vi "GUI_CapillaryDischarge.vi"() -> ()   [LabVIEW 2020]
uses:
  Shared/GUI_Template/GUI_master/tcp_new_data_event.ctl
  Shared/GUI_Template/GUI_master/tcp new data cluster.ctl
  timer.ctl
  <vilib>/Waveform/WDTOps.llb/WDT Waveform Duration DBL.vi
panel:
  in  "GUIdevice 10":string="SRS0"
  in  "time offsets":dbl[](array[numeric])=[0.0, 3e-09, 6e-08, 1.07e-07] format="%#_6p"
  in  "GUIdevice 9":string="Offsets-Timing"
  in  "Trigger on":bool caption="Discharge on"
  in  "GUIdevice 7":string="HeatHighlandT564"
  in  "Tab Control 2":T1(tab)
  out "all traces":waveform(dbl)[](graph)
  in  "value6::9":dbl=1.07e-07 caption="Dischage output" min=-9999999.0 max=9999999.0 step=1e-09 format="%#_6p"
  in  "value5::9":dbl=6e-08 caption="Dischage input" min=-9999999.0 max=9999999.0 step=1e-09 format="%#_6p"
  in  "value4::9":dbl=3e-09 caption="800nm diode" min=-9999999.0 max=9999999.0 step=1e-09 format="%#_6p"
  in  "value3::9":dbl caption="532nm diode" min=-9999999.0 max=9999999.0 step=1e-09 format="%#_6p"
  in  "Digitizer Traces":T2 caption="Digitizer Traces DAQ3 ch0 Timing diode Ch1 Discharge High"
  in  "Enable cap interlock move out":bool
  in  "Force button visibility":bool=TRUE
  in  "amplitude.Channel_C::10":dbl caption="Trigger voltage (0.1 off 1.2 on)" min=-3.0 max=4.0 step=1e-09 format="%#.2f"
  in  "Tab Control":enum32{"Settings for start button", "timeout"}(tab)
  in  "Set Pressure":dbl=30.0 caption="Timer 1 Value" min=0.0 max=100.0
  in  "Set Voltage":dbl=20.0 caption="Timer 1 Value" min=0.0 max=100.0
  in  "Start/Stop discharge":bool
  in  "Pressure Timeout":dbl=10.0 caption="Timer 1 Value" min=0.0 max=100.0
  in  "Voltage Timeout":dbl=10.0 caption="Timer 1 Value" min=0.0 max=100.0
  in  "slaveenable::1":bool
  out "pressure2::2":dbl caption="PDR UP (Torr)" min=-100.0 max=500.0
  in  "SlaveValue::1":dbl caption="Slave %" min=0.0 max=200.0
  out "Data.Channel 2::8":dbl caption="Flow UP (sccm)" min=0.0 max=1000.0
  out "Data.Channel 1::8":dbl caption="Flow Down (sccm)" min=0.0 max=1000.0
  in  "Data.Channel 2::1":dbl caption="PR4000 UP (Torr)" min=0.0 max=1000.0
  in  "GUIdevice 8":string="PL1-PresCtrl-Low2"
  out "Time Elasped Pressure 2":dbl
  out "Time Elasped Voltage 2":dbl
  out "Time Elasped Trig 2":dbl
  out "duration":dbl format="%.2p"
  in  "position::6":enum16{"out", "in", "Unknown"}(ring) caption="POSITION"
  in  "GUIdevice 6":string="PL1-Stage-Cap"
  in  "GUIdevice 5":string="LeCroy8104MS"
  in  "Simulate Trig Level":dbl
  out "Time Elasped Trig":dbl
  in  "Trigger Timeout":dbl=5.0 caption="Timer 1 Value" min=0.0 max=100.0
  in  "Set Trigger Level":dbl=4.0 caption="Timer 1 Value" min=0.0 max=100.0
  in  "GUIdevice 4":string="BellaSRS2"
  out "Discharge Status Msg":string
  out "Time Elasped Voltage":dbl
  in  "Simulate voltage":dbl
  in  "Simulate Pressure read":dbl
  in  "Simulate Pressure write":dbl
  in  "Simulate":bool
  out "Time Elasped Pressure":dbl
  out "pressure::2":dbl caption="PDR Down (Torr)" min=-100.0 max=500.0
  in  "voltage::3":dbl caption="Voltage (kV)" min=0.0 max=40.0
  out "Display Message":string
  in  "Data.Channel 1::1":dbl caption="PR4000 Down (Torr)" min=0.0 max=1000.0
  in  "GUIdevice 3":string="PL1-GlassmanHV"
  in  "GUIdevice 2":string="BELLA_PDR2000"
  in  "GUIdevice 1":string="PL1-PresCtrl-Low1"
  in  "stop":bool
  out "tcp data event":T3
  out "error IO 2":errorcluster
  # "CAPILLARY DISCHARGE CONTROL"
  # "CAPSTAGE"
  # "Check before moving capstage in\n1) pressure\n2) volts\n3) triggers\n4) discharge current"
  # "Diagnostics"
  # "Turn off procedure:\n1) reduce trigger level to 0.5\n2) reduce voltage to 0\n3) reduce pressure to 0"
  # "time offsets"
  # "start/stop needs testing. If doesn't work,\nuse controls on left"
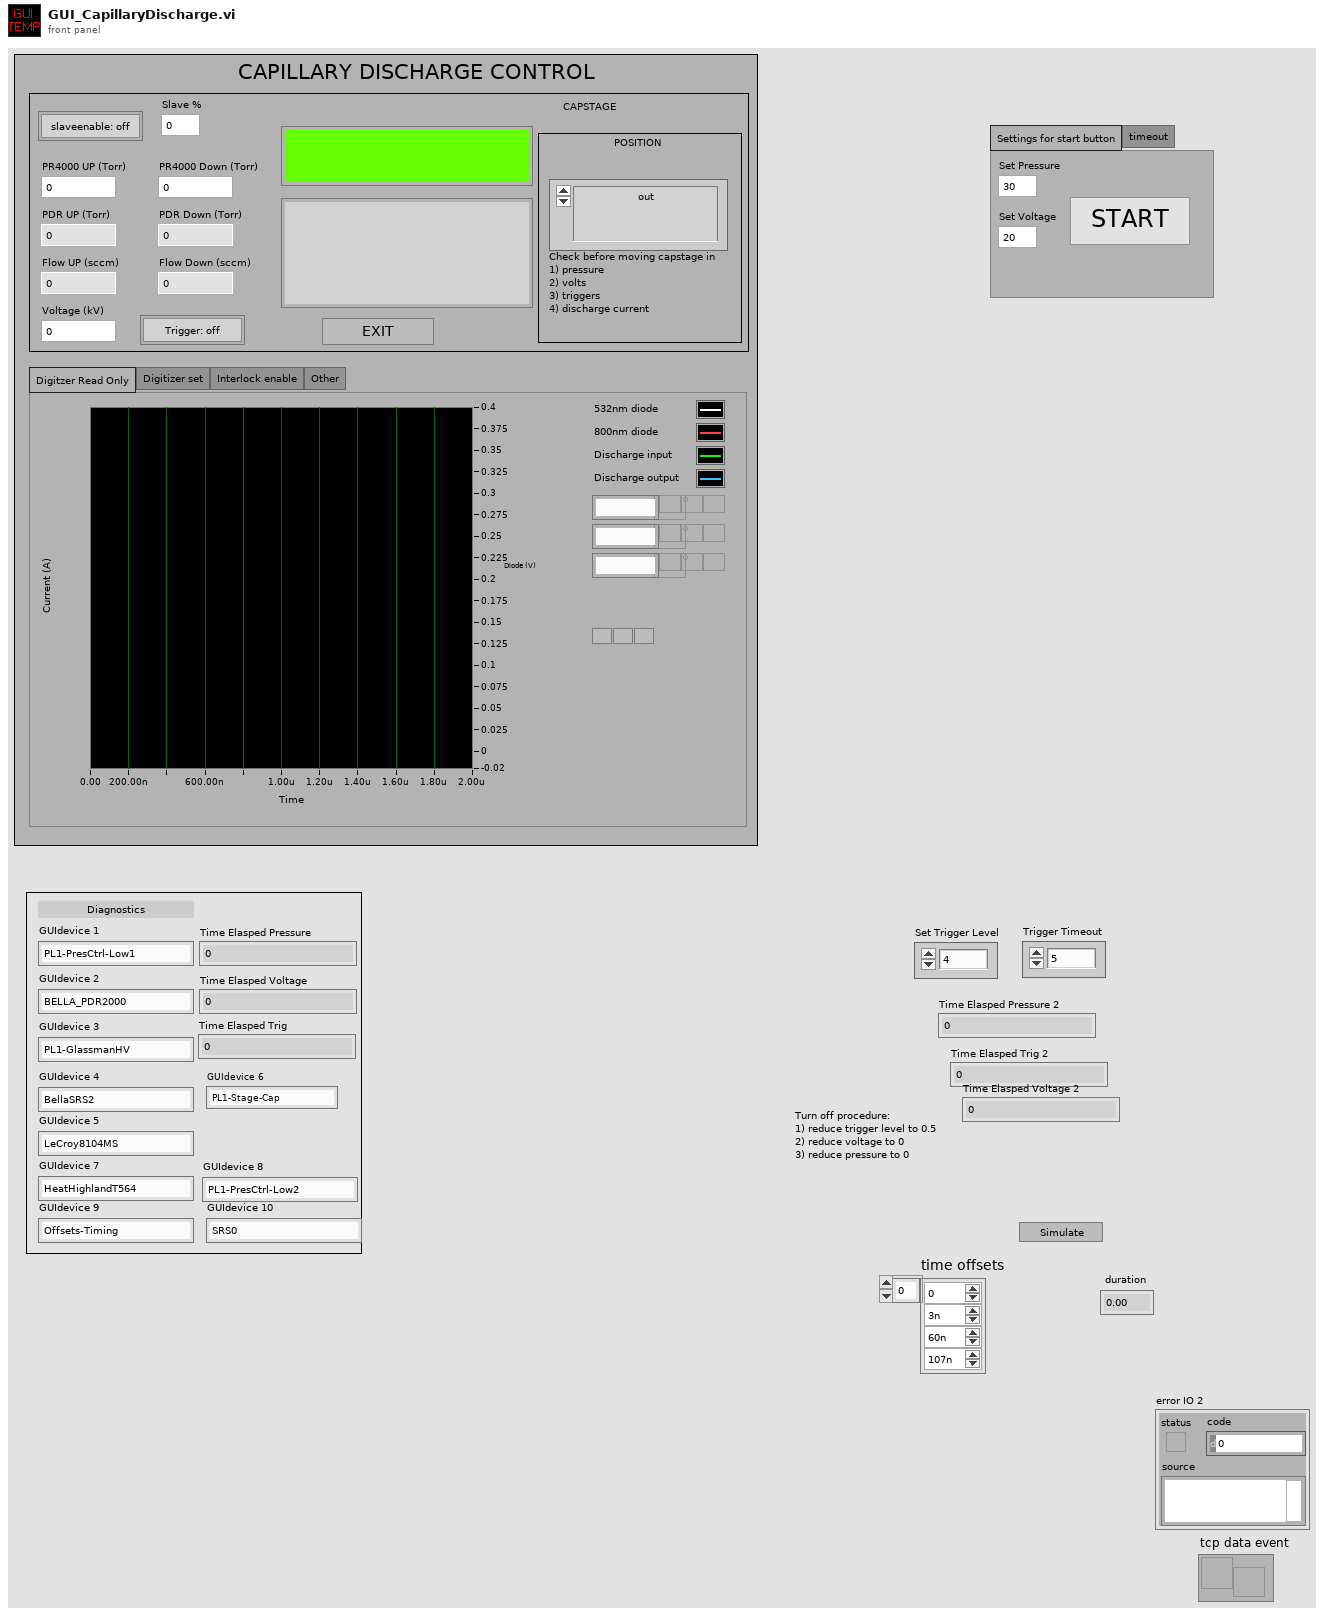
[diagram p1: front panel]
types:
  T1 = enum32{"Digitzer Read Only", "Digitizer set", "Interlock enable", "Other"}
  T2 = cluster{"Channel::5":enum16{"Channel0", "Channel1", "Channel2", "Channel3"}, "scopeTraceGUI::5":waveform(dbl)[]}
  T3 = typedef "tcp_new_data_event.ctl" = refnum<user-event>
  T4 = typedef "tcp new data cluster.ctl" = cluster{"EventEnum":enum16{"new data", "connection status update"}, "Device name":string}
  T5 = enum32{"invalid app kind", "Development System", "Run Time System", "Student Edition", "Embedded LabVIEW", "Evaluation", "Custom"}
  T6 = enum32{"Invalid", "Standard", "Closed", "Hidden", "Minimized", "Maximized"}
  T7 = typedef "timer.ctl" = enum16{"Start", "Read"}
  T8 = cluster{"Core":cluster{"Current VI Reference":refnum<vi>, "Close Panel on Exit?":bool}, "Pressure Timer":bool, "Voltage Timer":bool, "Pressure Timeout":dbl, "Voltage Timeout":dbl, "Display Message":string, "Simulate":bool, "Trigger Timeout":dbl, "Trigger Timer":bool, "Discharge Status Msg":string, "scopeTraceGUI::5":waveform(dbl)[], "scopeTraceGUI::7":waveform(dbl)[]}
  T9 = cluster{"Current VI Reference":refnum<vi>, "Close Panel on Exit?":bool}
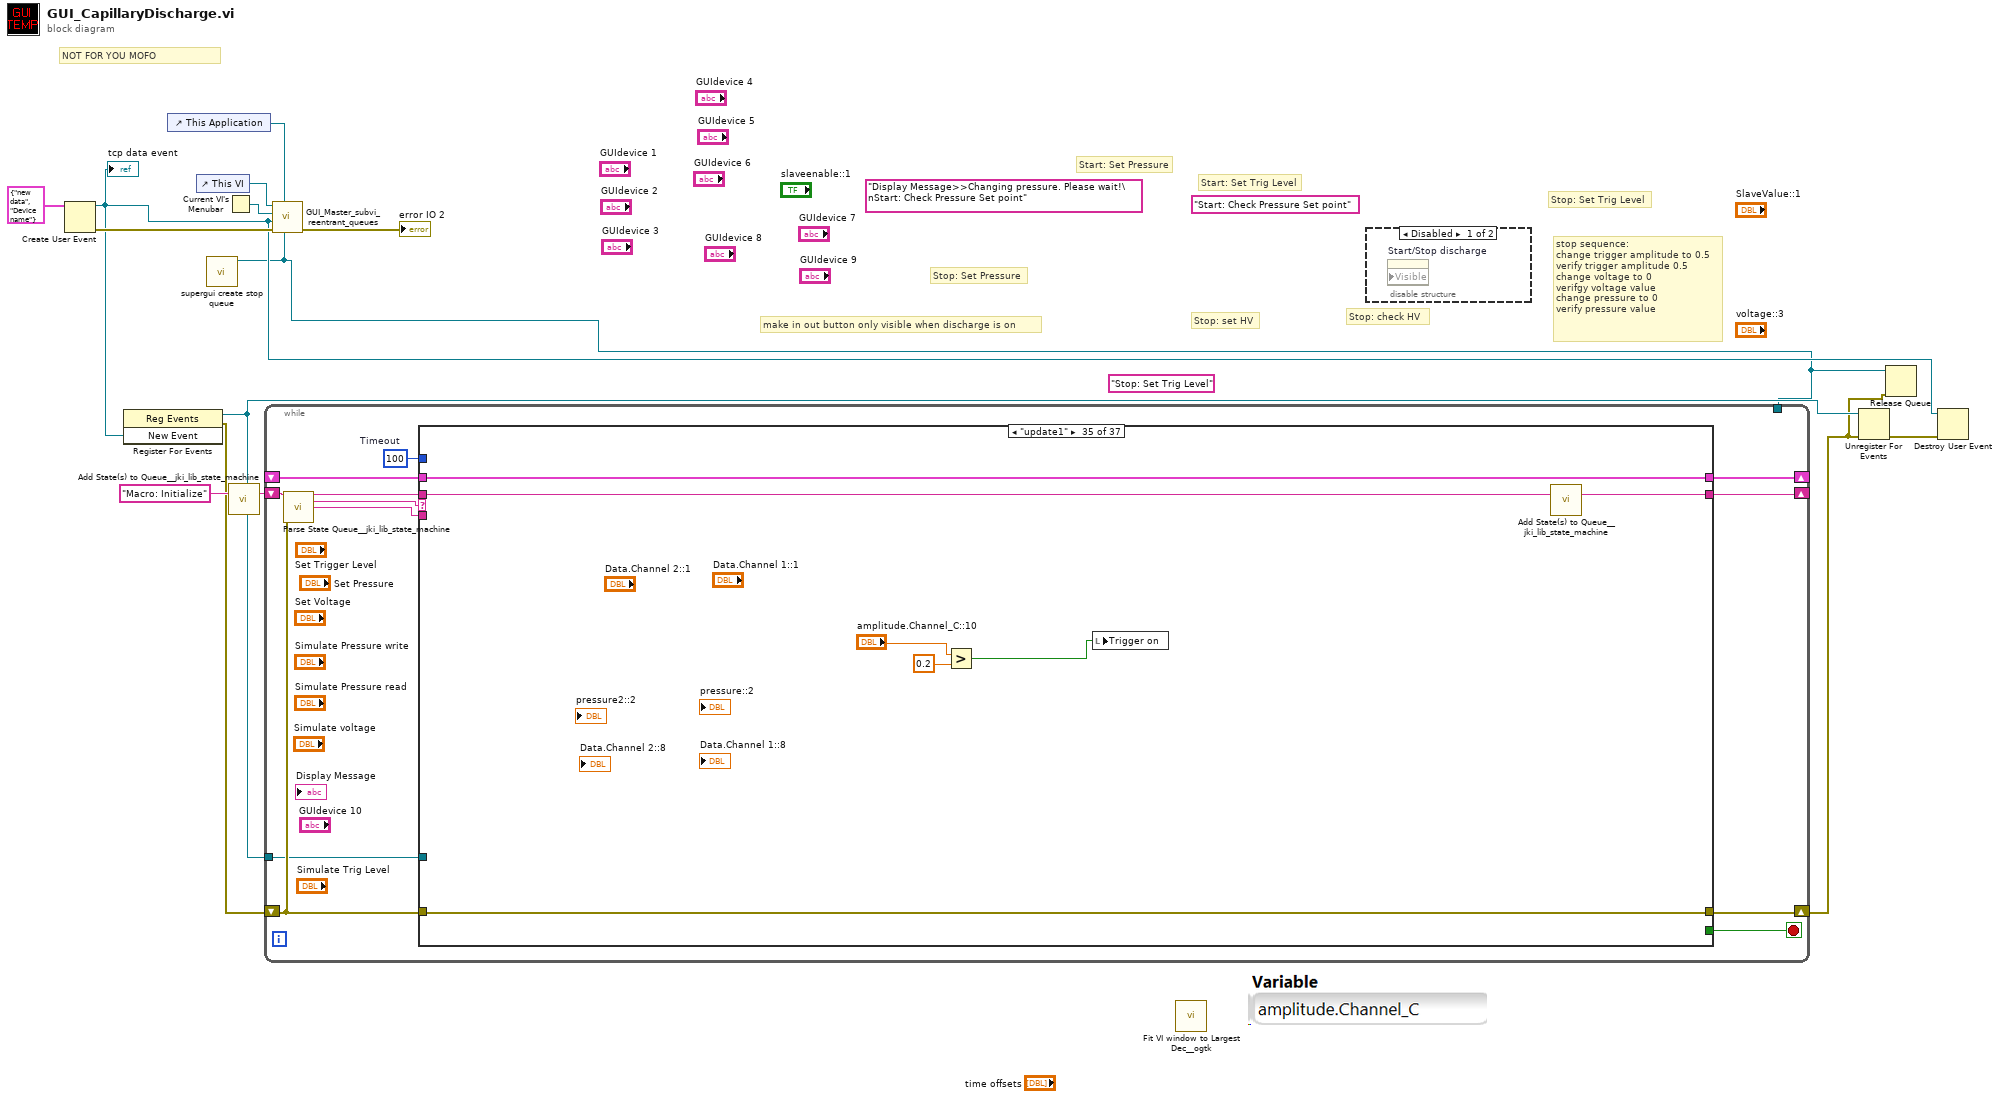
[diagram p0: block diagram]
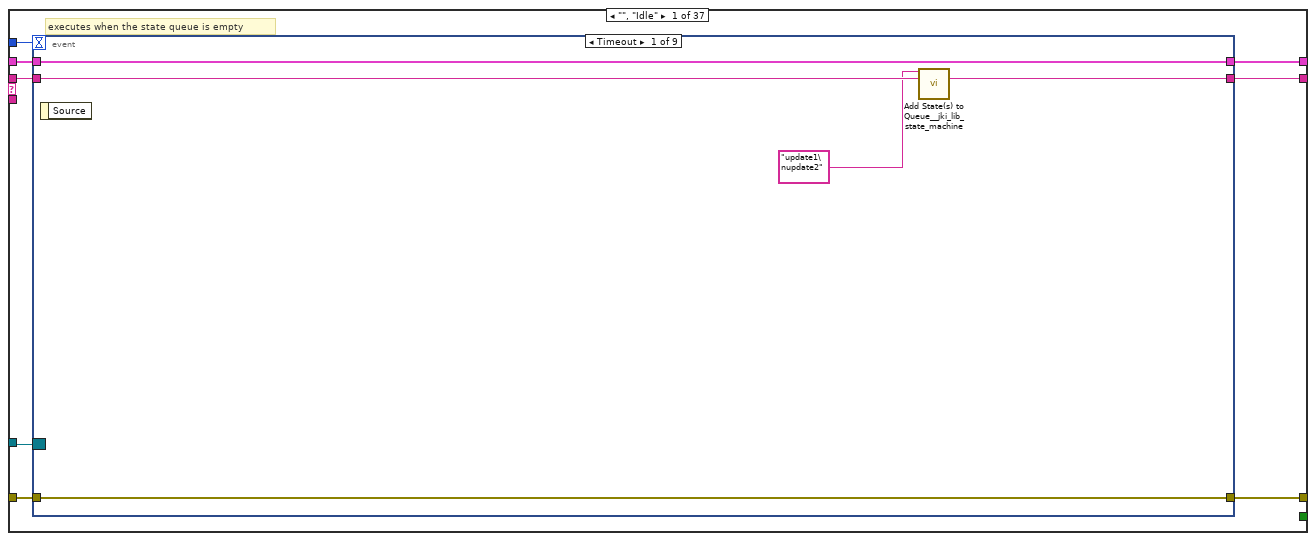
[diagram p3: hidden frame]
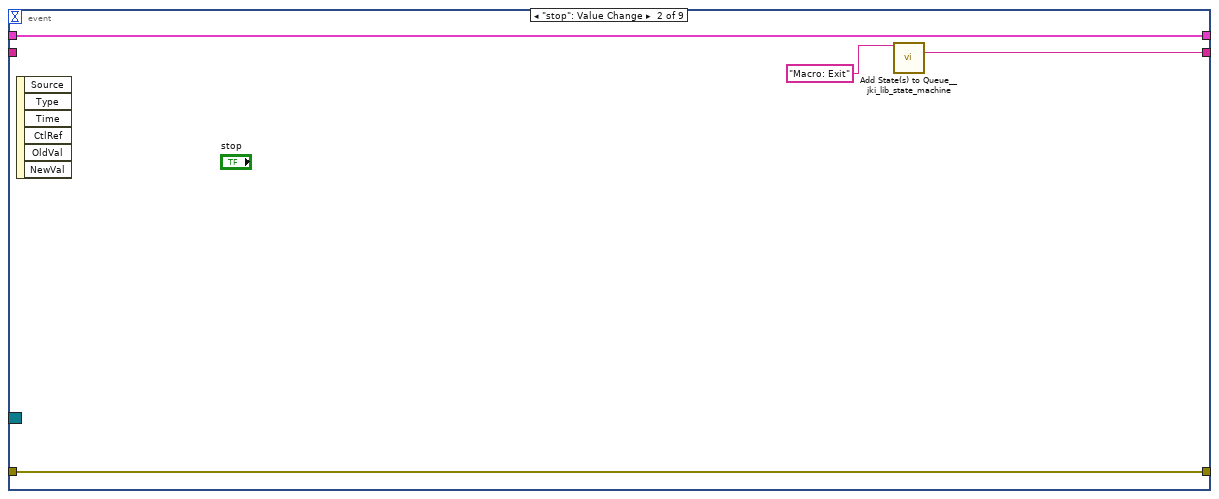
[diagram p4: hidden frame]
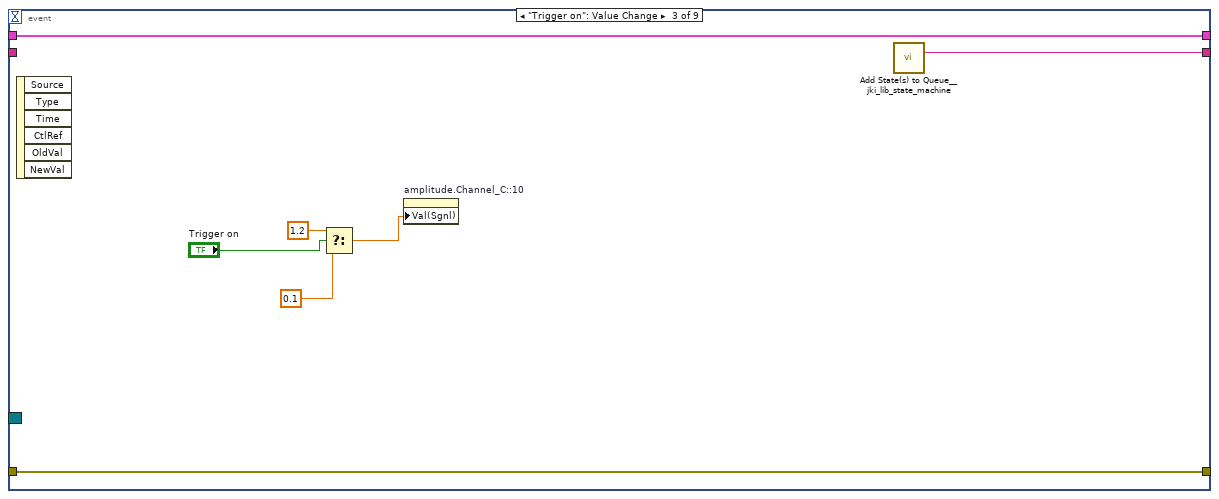
[diagram p5: hidden frame]
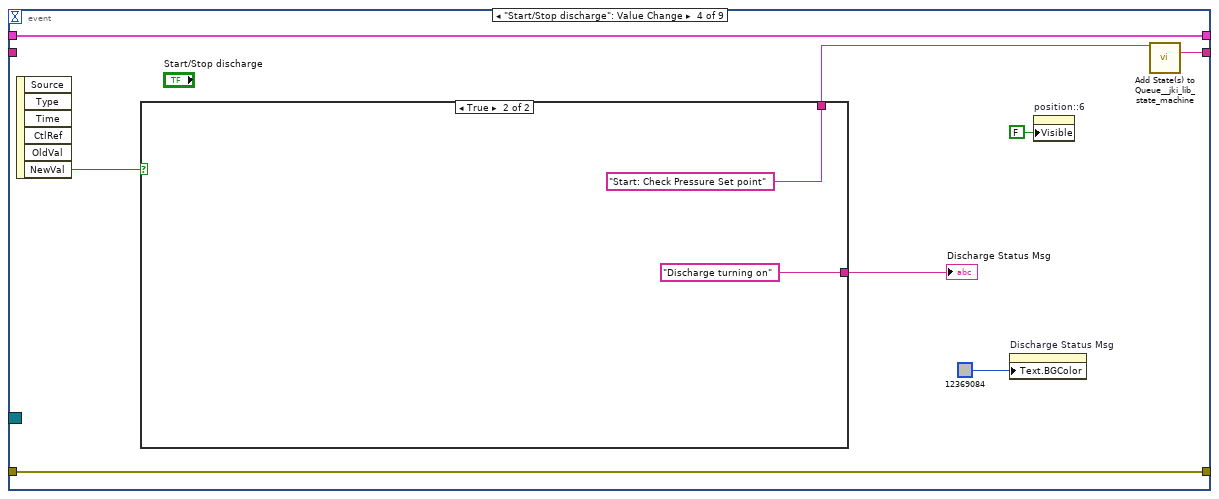
[diagram p6: hidden frame]
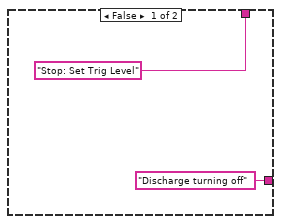
[diagram p7: hidden frame]
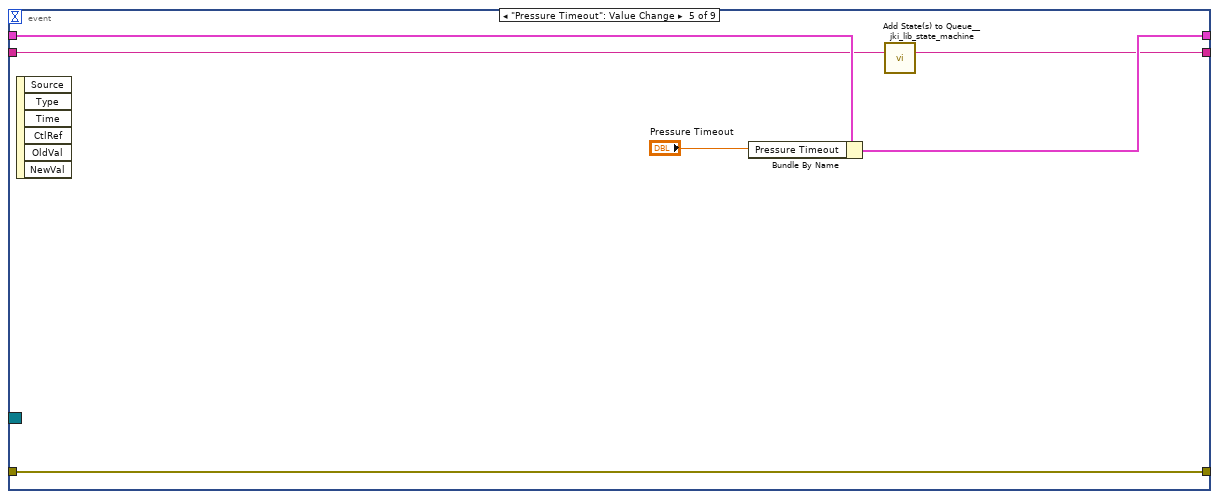
[diagram p8: hidden frame]
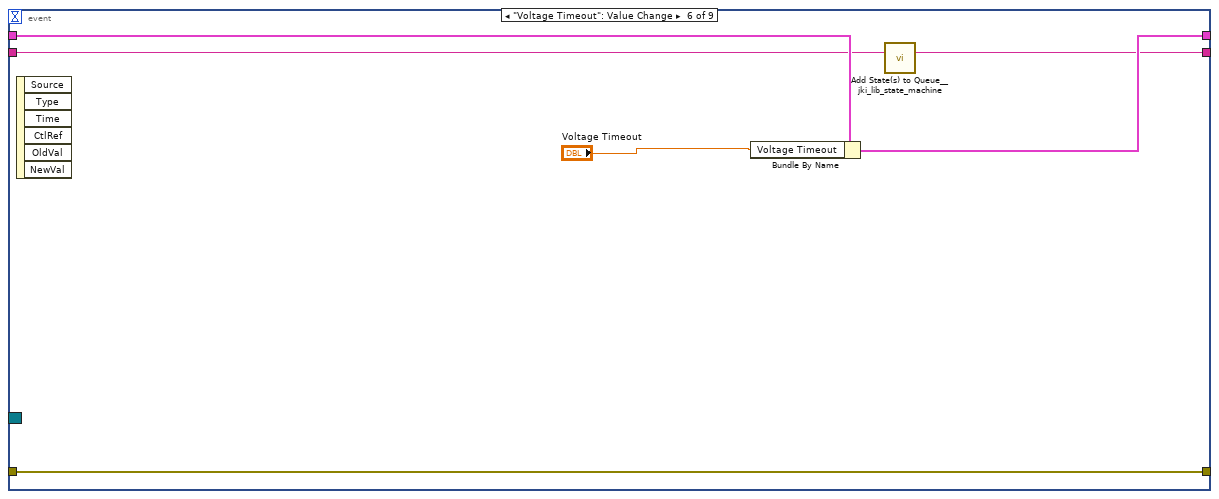
[diagram p9: hidden frame]
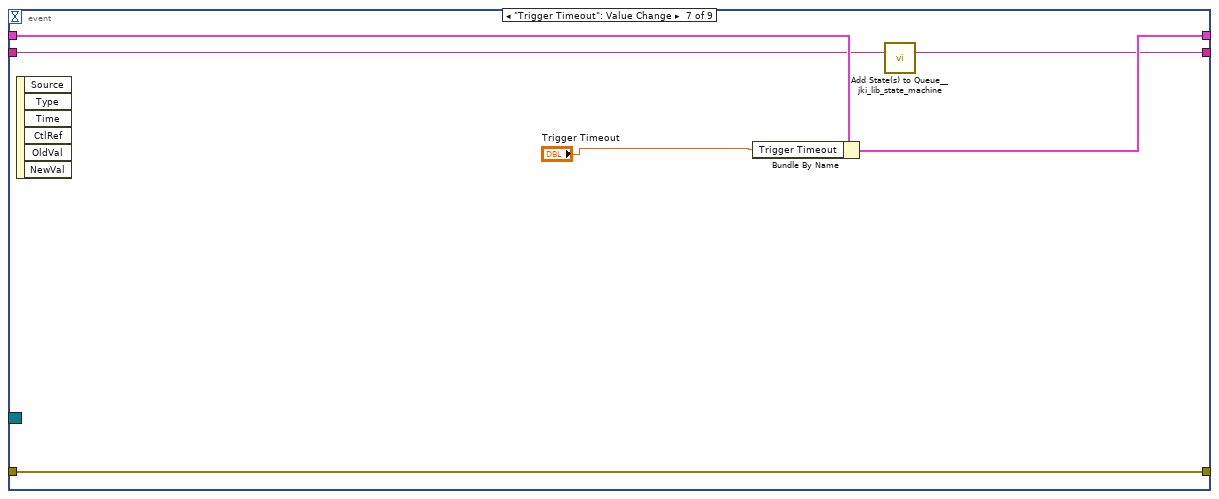
[diagram p10: hidden frame]
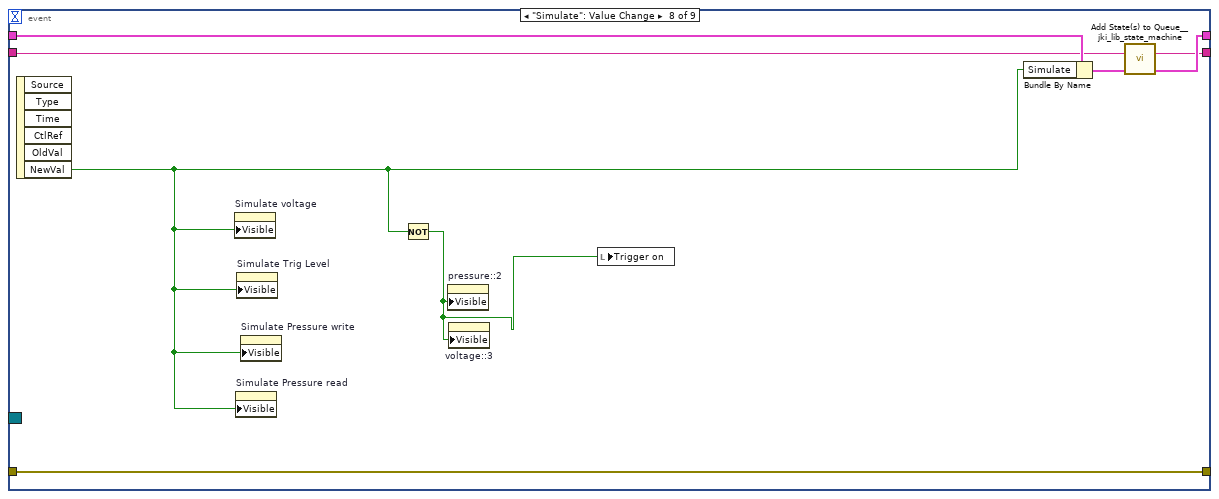
[diagram p11: hidden frame]
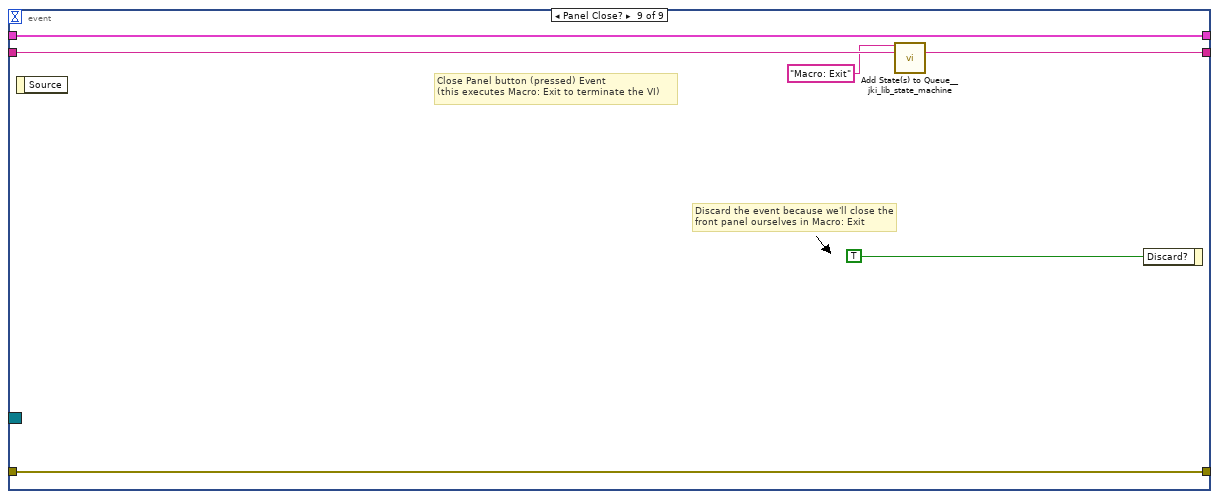
[diagram p12: hidden frame]
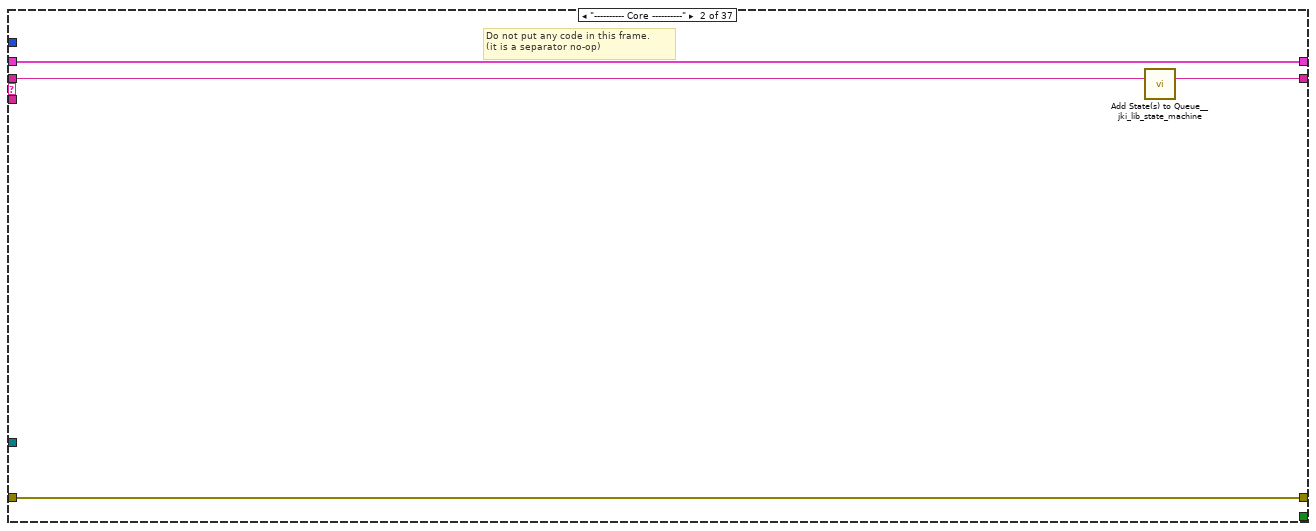
[diagram p13: hidden frame]
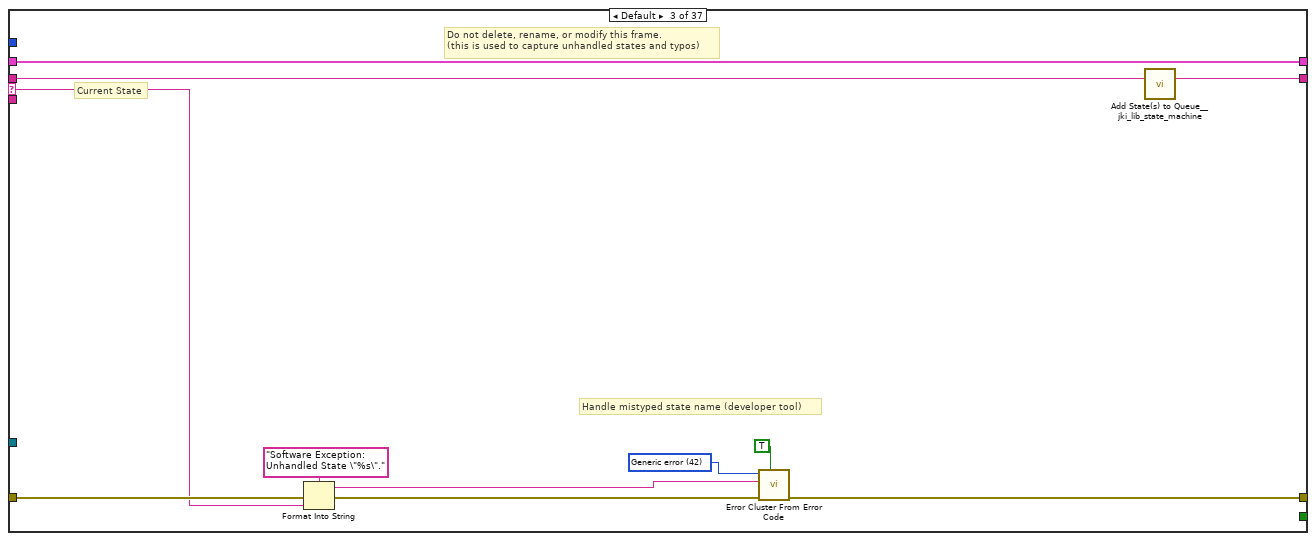
[diagram p14: hidden frame]
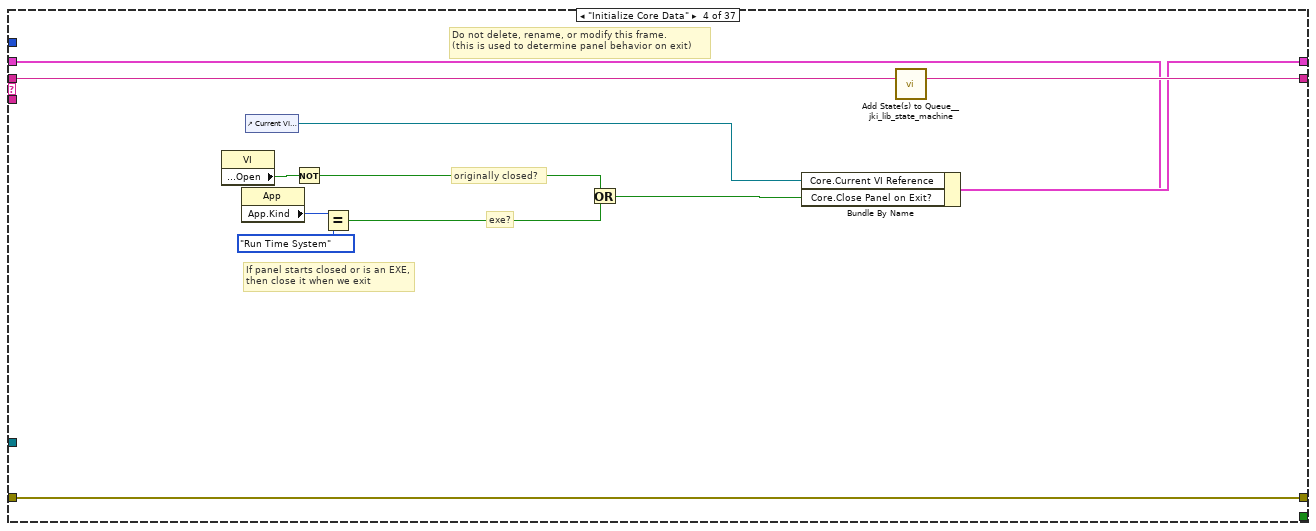
[diagram p15: hidden frame]
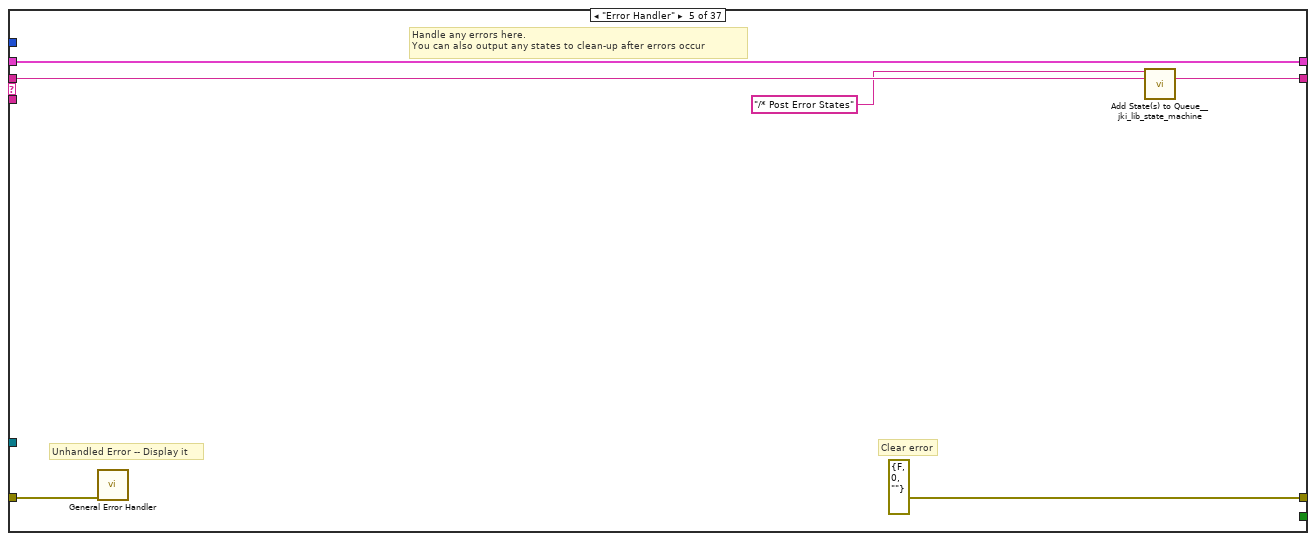
[diagram p16: hidden frame]
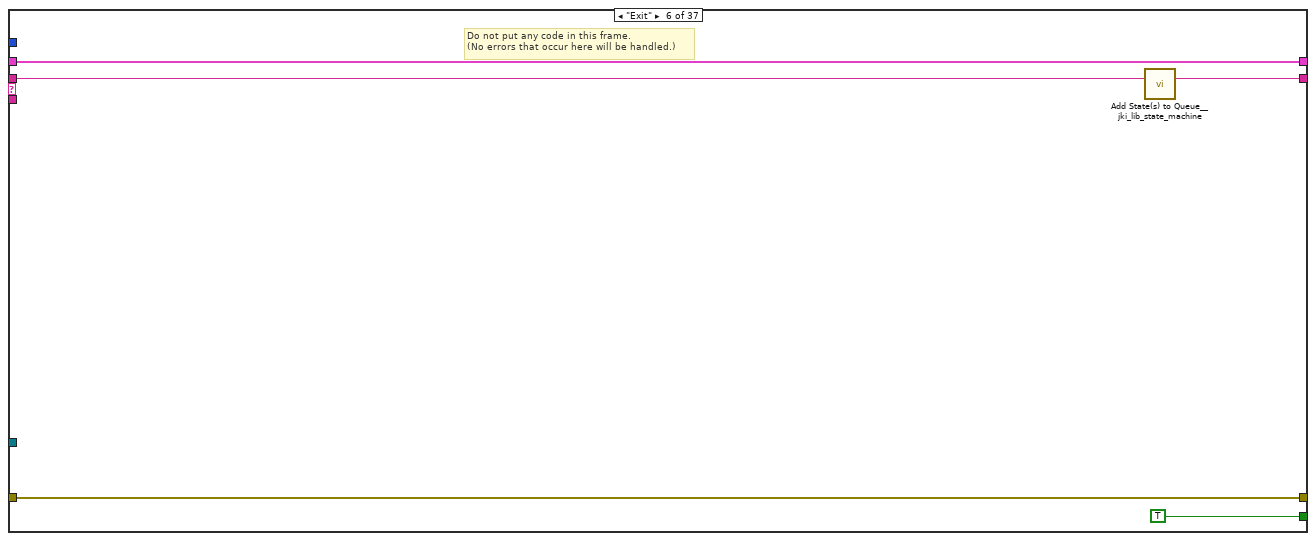
[diagram p17: hidden frame]
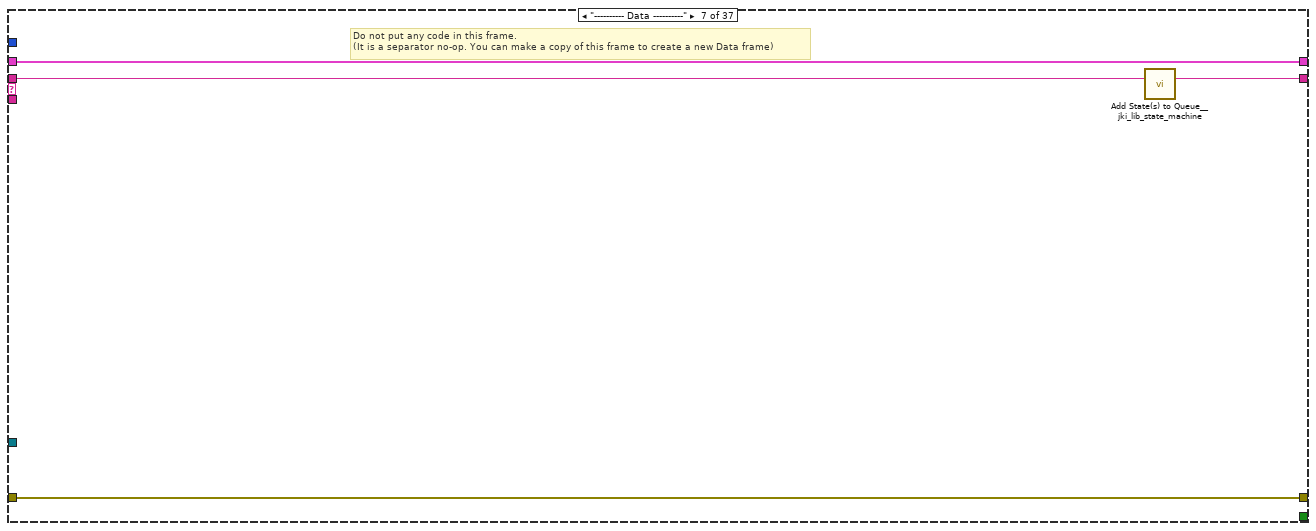
[diagram p18: hidden frame]
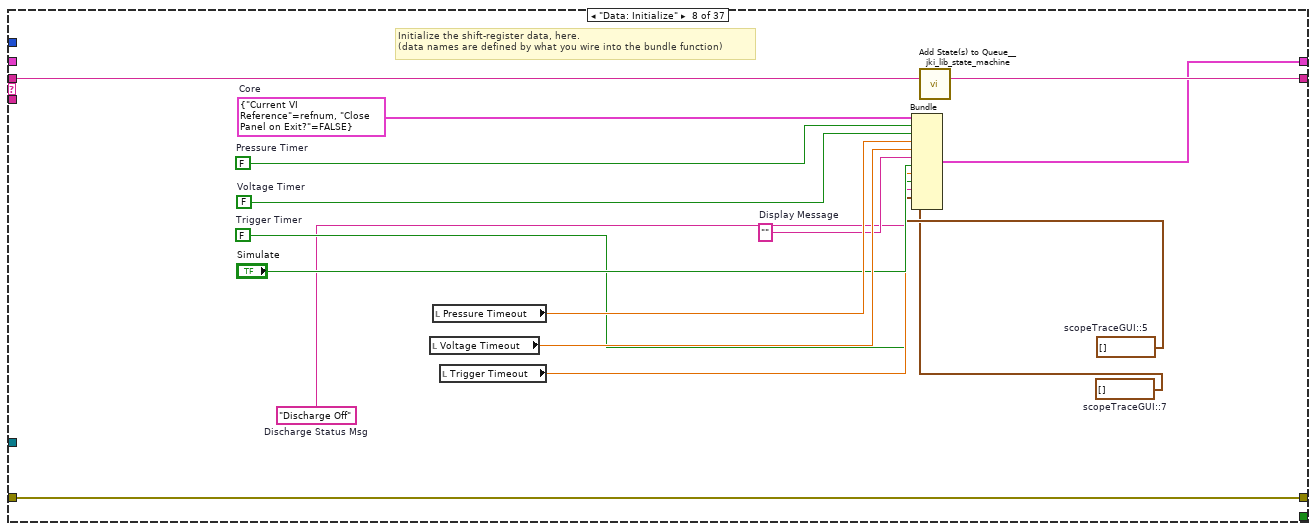
[diagram p19: hidden frame]
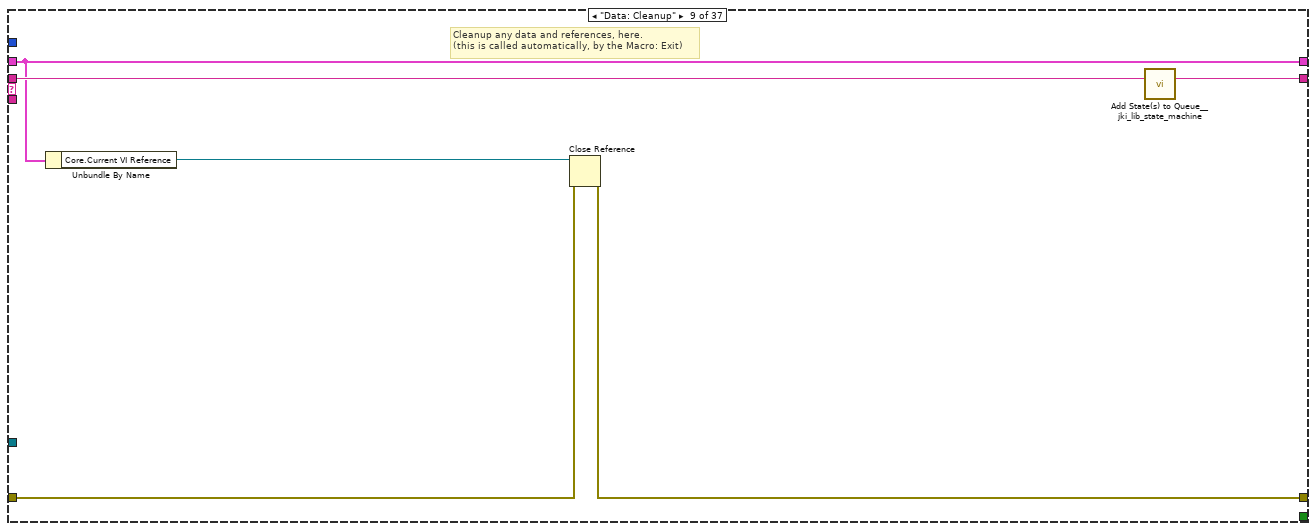
[diagram p20: hidden frame]
diagram:
  (unwired) "Stop: Set Trig Level"
  (unwired) "Start: Check Pressure Set point"
  (unwired) "Display Message>>Changing pressure. Please wait!\nStart: Check Pressure Set point" ("State(s) in Front (\"\")")
  # "make in out button only visible when discharge is on"
  # "Stop: Set Pressure"
  # "Stop: check HV"
  # "Stop: set HV"
  # "Stop: Set Trig Level"
  # "stop sequence:\nchange trigger amplitude to 0.5\nverify trigger amplitude 0.5\nchange voltage to 0\nverifgy voltage value\nchange pressure to 0\nverify pressure value"
  # "Start: Set Pressure"
  # "Start: Set Trig Level"
  # "NOT FOR YOU MOFO"
  n1 = Create User Event(user event datatype=T4 {"EventEnum"=enum."new data", "Device name"="Device name"} ("New Event")) -> (user event=w8:refnum<user-event>, error out=w10:errorcluster)  [unwired: 1 in]
  "tcp data event" <- w8
  n2 = register-events(w8) -> (reference out=w4:refnum<event-registration>, error out=w5:errorcluster)  [unwired: 2 in]
  n3 = control-ref of="This Application"() -> (w9:refnum<vi>)
  n4 = control-ref of="This VI"() -> (w13:refnum<vi>)
  n5 = call "supergui create stop queue.vi"() -> ("STOP Queue out"=w3:refnum<queue>)  [unwired: 11 in]
  n6 = Current VI's Menubar() -> (w12:refnum<k9>)
  n7 = call <vilib>:"Add State(s) to Queue__jki_lib_state_machine.vi"("State(s) in (\"\")"="Macro: Initialize") -> ("States Out"=w7:string)  [unwired: 14 in]
  n8 = while "JKI - String-Based Queued State Machine (Basic) v1.0" {
    shift-right: [w19] -> _
    shift-left: _ -> [w18]
    shift-right: [w22] -> w1
    shift-left: w5 -> [w16]
    shift-right: [w21] -> _
    shift-left: w7 -> [w23]
    tunnel: w4 -> [w15]
    tunnel: w3 -> [_]
    stop <- w20 stop-if-true
    w17 = 100  # Timeout
    n9 = call <vilib>:"Parse State Queue__jki_lib_state_machine.vi"("State Queue"=w23, "Error In (no error)"=w16) -> ("Remaining States"=w25:string, "Current State"=w26:string, "Arguments"=w24:string)  [unwired: 11 in]
    n10 = case shown="\"update1\"" w26 {
      selector: w26 -> [_ _ w98 _ _ _ _ _ _ _ _ _ _ _ _ _ _ _ _ _ _ _ _ _ _ _ _ _ _ _ _ _ _ _ _ _ _]
      tunnel: w25 -> [w34 w97 w102 w120 w126 w131 w135 w151 w157 w161 w167 w177 w188 w214 w219 w229 w233 w242 w277 w305 w318 w329 w367 w395 w409 w417 w440 w462 w473 w485 w491 w497 w504 w540 w581 w585 w599]
      tunnel: w24 -> [_ _ _ _ _ _ _ _ _ _ _ w172 w182 _ _ _ _ _ _ _ _ _ _ _ _ _ _ _ _ _ _ _ w500 _ _ _ _]
      tunnel: w18 -> [w32 w94 w100 w111 w123 w129 w132 _ w152 w158 w163 w175 w184 w211 w216 w227 w230 w237 w272 w299 w312 w322 w361 w389 w403 w416 w439 w460 w471 w482 w488 w494 w498 w507 w578 w582 w594]
      tunnel: [w31 w95 w104 w117 errorcluster {"status"=FALSE, "code"=0, "source"=""} ("error out") w128 w133 w148 w153 w159 w165 w173 w185 w212 w217 w220 w231 w240 w275 w303 w316 w327 w365 w393 w407 w413 w436 w458 w469 w483 w489 w495 w502 w538 w579 w583 w586] -> w22
      tunnel: w16 -> [w30 w95 w103 w117 w122 w128 w133 w148 w154 w159 w165 w174 w186 w212 w217 w220 w231 w240 w275 w303 w316 w327 w365 w393 w407 w413 w436 w458 w469 w483 w489 w495 w502 w538 w579 w583 w587]
      tunnel: [w33 w96 w101 w119 w125 w130 w134 w150 w156 w160 w166 w176 w187 w213 w218 w228 w232 w241 w276 w304 w317 w328 w366 w394 w408 w414 w437 w461 w472 w484 w490 w496 w503 w539 w580 w584 w598] -> w21
      tunnel: [_ _ _ _ _ TRUE _ _ _ _ _ _ _ _ _ _ _ _ _ _ _ _ _ _ _ _ _ _ _ _ _ _ _ _ _ _ _] -> w20
      tunnel: [w29 w94 w100 w118 w123 w129 w132 w149 w152 w158 w163 w175 w184 w211 w216 w227 w230 w236 w271 w301 w314 w321 w360 w391 w405 w415 w438 w459 w470 w481 w487 w493 w498 w507 w578 w582 w596] -> w19
      tunnel: w17 -> [w28 _ _ _ _ _ _ _ _ _ _ _ _ _ _ _ _ _ _ _ _ _ _ _ _ _ _ _ _ _ _ _ _ _ _ _ _]
      tunnel: w15 -> [w27 _ _ _ _ _ _ _ _ _ _ _ _ _ _ _ _ _ _ _ _ _ _ _ _ _ _ _ _ _ _ _ _ _ _ _ _]
      frame "", "Idle" {
        # "executes when the state queue is empty"
        n11 = event shown="[0] Timeout" {
          selector: w27 -> [_ _ _ _ _ _ _ _ _]
          dyn-events: _ -> [_ _ _ _ _ _ _ _ _]
          timeout: w28 -> [_ _ _ _ _ _ _ _ _]
          tunnel: w34 -> [w39 _ _ _ w64 w71 w77 w83 w93]
          tunnel: [w38 w41 w49 w57 w63 w70 w76 w84 w92] -> w33
          tunnel: w32 -> [w36 w43 w50 w58 w67 w73 w79 w87 w90]
          tunnel: [w37 w40 w48 w56 w68 w74 w80 w85 w91] -> w31
          tunnel: w30 -> [w37 w40 w48 w56 w68 w74 w80 w85 w91]
          tunnel: [w36 w43 w50 w58 w66 w72 w78 w86 w90] -> w29
          event Timeout {
            n12 = event-data() -> ()  [unwired: 1 in, 1 out]
            n13 = call <vilib>:"Add State(s) to Queue__jki_lib_state_machine.vi"("State(s) in Front (\"\")"="update1\nupdate2" ("State(s) in Front (\"\")"), "State(s) in (\"\")"=w39) -> ("States Out"=w38:string)  [unwired: 13 in]
          }
          event "stop": Value Change {
            n14 = event-data() -> ()  [unwired: 1 in, 6 out]
            n15 = call <vilib>:"Add State(s) to Queue__jki_lib_state_machine.vi"("State(s) in Front (\"\")"="Macro: Exit") -> ("States Out"=w41:string)  [unwired: 14 in]
          }
          event "Trigger on": Value Change {
            n16 = event-data() -> ()  [unwired: 1 in, 6 out]
            n17 = Select(t=1.2, s="Trigger on", f=0.1 ("t")) -> (s? t:f=w44:dbl)
            n18 = property on="amplitude.Channel_C::10" class="DigNum (strict)"("Val(Sgnl)"=w44) -> ()  [unwired: 2 in, 2 out]
            n19 = call <vilib>:"Add State(s) to Queue__jki_lib_state_machine.vi"() -> ("States Out"=w49:string)  [unwired: 15 in]
          }
          event "Start/Stop discharge": Value Change {
            n20 = event-data() -> ("NewVal"=w55:bool)  [unwired: 1 in, 5 out]
            n21 = case shown="True" w55 {
              tunnel: ["Stop: Set Trig Level" "Start: Check Pressure Set point"] -> w54
              tunnel: ["Discharge turning off" ("Discharge Status Msg") "Discharge turning on" ("Discharge Status Msg")] -> w52
              frame False {
              }
              frame True {
              }
            }
            "Discharge Status Msg" <- w52
            n22 = property on="Discharge Status Msg" class="Str"("Text.BGColor"=u32 12369084) -> ()  [unwired: 2 in, 2 out]
            n23 = property on="position::6" class="Enum (strict)"("Visible"=FALSE) -> ()  [unwired: 2 in, 2 out]
            n24 = call <vilib>:"Add State(s) to Queue__jki_lib_state_machine.vi"("State(s) in Front (\"\")"=w54) -> ("States Out"=w57:string)  [unwired: 14 in]
          }
          event "Pressure Timeout": Value Change {
            n25 = event-data() -> ()  [unwired: 1 in, 6 out]
            n26 = Bundle By Name(cluster=w67, "Pressure Timeout"="Pressure Timeout") -> (w66:T8)
            n27 = call <vilib>:"Add State(s) to Queue__jki_lib_state_machine.vi"("State(s) in (\"\")"=w64) -> ("States Out"=w63:string)  [unwired: 14 in]
          }
          event "Voltage Timeout": Value Change {
            n28 = event-data() -> ()  [unwired: 1 in, 6 out]
            n29 = Bundle By Name(cluster=w73, "Voltage Timeout"="Voltage Timeout") -> (w72:T8)
            n30 = call <vilib>:"Add State(s) to Queue__jki_lib_state_machine.vi"("State(s) in (\"\")"=w71) -> ("States Out"=w70:string)  [unwired: 14 in]
          }
          event "Trigger Timeout": Value Change {
            n31 = event-data() -> ()  [unwired: 1 in, 6 out]
            n32 = Bundle By Name(cluster=w79, "Trigger Timeout"="Trigger Timeout") -> (w78:T8)
            n33 = call <vilib>:"Add State(s) to Queue__jki_lib_state_machine.vi"("State(s) in (\"\")"=w77) -> ("States Out"=w76:string)  [unwired: 14 in]
          }
          event "Simulate": Value Change {
            n34 = event-data() -> ("NewVal"=w82:bool)  [unwired: 1 in, 5 out]
            n35 = property on="Simulate voltage" class="DigNum (strict)"("Visible"=w82) -> ()  [unwired: 2 in, 2 out]
            n36 = property on="Simulate Pressure read" class="DigNum (strict)"("Visible"=w82) -> ()  [unwired: 2 in, 2 out]
            n37 = property on="Simulate Trig Level" class="DigNum (strict)"("Visible"=w82) -> ()  [unwired: 2 in, 2 out]
            n38 = property on="Simulate Pressure write" class="DigNum (strict)"("Visible"=w82) -> ()  [unwired: 2 in, 2 out]
            n39 = Not(x=w82) -> (.not. x?=w81:bool)
            n40 = property on="pressure::2" class="DigNum (strict)"("Visible"=w81) -> ()  [unwired: 2 in, 2 out]
            n41 = property on="voltage::3" class="DigNum (strict)"("Visible"=w81) -> ()  [unwired: 2 in, 2 out]
            n42 = local write "Trigger on"(w81) -> ()
            n43 = Bundle By Name(cluster=w87, "Simulate"=w82) -> (w86:T8)
            n44 = call <vilib>:"Add State(s) to Queue__jki_lib_state_machine.vi"("State(s) in (\"\")"=w83) -> ("States Out"=w84:string)  [unwired: 14 in]
          }
          event Panel Close? {
            # "Discard the event because we'll close the front panel ourselves in Macro: Exit"
            # "Close Panel button (pressed) Event\n(this executes Macro: Exit to terminate the VI)"
            n45 = event-data() -> ()  [unwired: 1 in, 1 out]
            n46 = call <vilib>:"Add State(s) to Queue__jki_lib_state_machine.vi"("State(s) in Front (\"\")"="Macro: Exit", "State(s) in (\"\")"=w93) -> ("States Out"=w92:string)  [unwired: 13 in]
            n47 = event-data("Discard?"=TRUE) -> ()  [unwired: 1 in, 1 out]
          }
        }
      }
      frame "---------- Core ----------" {
        # "Do not put any code in this frame.\n(it is a separator no-op)"
        n48 = call <vilib>:"Add State(s) to Queue__jki_lib_state_machine.vi"("State(s) in (\"\")"=w97) -> ("States Out"=w96:string)  [unwired: 14 in]
      }
      frame Default {
        w107 = 42 items=["No error", "Argument error", "Memory is full", "Out of zone", "End of file", "File already open", "Generic file I/O error", "File not found", "File permission error", "Disk is full", "Duplicate path", "Too many files open", "System feature not enabled", "Resource file not found", "Cannot add resource", "Resource not found", "Image not found", "Image memory error", "Pen does not exist", "Config type invalid", "Config token not found", "Config parse error", "Config memory error", "Bad external code format", "Bad external code offset", "External code not present", "Null window", "Destroy window error", "Null menu", "Print aborted", "Bad print record", "Print driver error", "Windows error during printing", "Memory error during printing", "Print dialog error", "Generic print error", "Invalid device refnum", "Device not found", "Device parameter error", "Device unit error", "Cannot open device", "Device call aborted", "Generic error", "Cancelled by user", "Object ID too low", "Object ID too high", "Object not in heap", "Unknown heap", "Unknown object (invalid DefProc)", "Unknown object (DefProc not in table)", "Message out of range", "Invalid (null) method", "Unknown message", "Manager call not supported", "Bad address", "Network operation in progress", "Network operation timed out", "Connection is busy", "Network attribute not supported", "Network error", "Address in use", "System out of memory", "Connection aborted", "Connection refused", "Not connected", "Already connected", "Connection closed", "Initialization error (interapplication manager)", "Bad occurrence", "Wait on unbound occurrence handler", "Occurrence queue overflow", "Datalog type conflict", "Unused", "Unrecognized type (interapplication manager)", "Memory corrupt", "Failed to make temporary DLL", "Old CIN version", "Drag socket not found", "Failed to load drop-object", "Failed to register OLE object", "Failed to release OLE object", "Format specifier type mismatch", "Unknown format specifier", "Too few format specifiers", "Too many format specifiers", "Scan failed", "Newer CIN version", "Error converting to variant", "Runtime menu error", "Password tampered", "Variant attribute not found", "Incompatible variant data type", "Event data is not available", "Event Store is not present", "Occurrence is not found", "Event Queue is not created", "Event info is not available", "Refnum passed is NULL", "Error retrieving Class GUID", "Error retrieving CoClass GUID", "Error retrieving TypeLib GUID.", "Bad built application magic bytes.", "Specific driver is different from the specific driver associated with the Logical Name.", "There is no session opened to the class driver.", "Max Error", "MAX - Error with config objects", "MAX - Error loading configuration", "MAX - Group not supported"]
        # "Current State"
        # "Do not delete, rename, or modify this frame.\n(this is used to capture unhandled states and typos)"
        # "Handle mistyped state name (developer tool)"
        n49 = Format Into String(format string="Software Exception: Unhandled State \"%s\"." ("message"), error in=w103, w98) -> (resulting string=w106:string, error out=w105:errorcluster)  [unwired: 1 in]
        n50 = call <vilib>:"Error Cluster From Error Code.vi"("show call chain? (False)"=TRUE, "error in (no error)"=w105, "error message (\"\")"=w106, "error code (0)"=w107) -> ("error out"=w104:errorcluster)  [unwired: 5 in]
        n51 = call <vilib>:"Add State(s) to Queue__jki_lib_state_machine.vi"("State(s) in (\"\")"=w102) -> ("States Out"=w101:string)  [unwired: 14 in]
      }
      frame "Initialize Core Data" {
        # "Do not delete, rename, or modify this frame.\n(this is used to determine panel behavior on exit)"
        # "originally closed?"
        # "exe?"
        # "If panel starts closed or is an EXE, then close it when we exit"
        n52 = property class="VI"() -> ("Front Panel.Open"=w116:bool)  [unwired: 2 in, 2 out]
        n53 = property class="App"() -> ("App.Kind"=w115:T5)  [unwired: 2 in, 2 out]
        n54 = control-ref of="Current VI Reference"() -> (w109:refnum<vi>)
        n55 = Not(x=w116) -> (.not. x?=w113:bool)
        n56 = Equal?(x=w115, y=T5."Run Time System" ("Application:Kind")) -> (x = y?=w112:bool)
        n57 = Or(x=w113, y=w112) -> (x .or. y?=w110:bool)
        n58 = Bundle By Name(cluster=w111, "Core.Current VI Reference"=w109, "Core.Close Panel on Exit?"=w110) -> (w118:T8)
        n59 = call <vilib>:"Add State(s) to Queue__jki_lib_state_machine.vi"("State(s) in (\"\")"=w120) -> ("States Out"=w119:string)  [unwired: 14 in]
      }
      frame "Error Handler" {
        # "Unhandled Error -- Display it"
        # "Handle any errors here.\nYou can also output any states to clean-up after errors occur"
        # "Clear error"
        n60 = call <vilib>:"General Error Handler.vi"("error in (no error)"=w122) -> ()  [unwired: 10 in, 5 out]
        n61 = call <vilib>:"Add State(s) to Queue__jki_lib_state_machine.vi"("State(s) in Front (\"\")"="/* Post Error States", "State(s) in (\"\")"=w126) -> ("States Out"=w125:string)  [unwired: 13 in]
      }
      frame "Exit" {
        # "Do not put any code in this frame.\n(No errors that occur here will be handled.)"
        n62 = call <vilib>:"Add State(s) to Queue__jki_lib_state_machine.vi"("State(s) in (\"\")"=w131) -> ("States Out"=w130:string)  [unwired: 14 in]
      }
      frame "---------- Data ----------" {
        # "Do not put any code in this frame.\n(It is a separator no-op. You can make a copy of this frame to create a new Data frame)"
        n63 = call <vilib>:"Add State(s) to Queue__jki_lib_state_machine.vi"("State(s) in (\"\")"=w135) -> ("States Out"=w134:string)  [unwired: 14 in]
      }
      frame "Data: Initialize" {
        w136 = waveform(dbl)[] []  # scopeTraceGUI::7
        w137 = waveform(dbl)[] []  # scopeTraceGUI::5
        w138 = "Discharge Off"  # Discharge Status Msg
        w139 = FALSE  # Trigger Timer
        w142 = ""  # Display Message
        w145 = FALSE  # Voltage Timer
        w146 = T9 {"Current VI Reference"=refnum, "Close Panel on Exit?"=FALSE}  # Core
        w147 = FALSE  # Pressure Timer
        # "Initialize the shift-register data, here.\n(data names are defined by what you wire into the bundle function)"
        n64 = local read "Voltage Timeout"() -> (w143:dbl)
        n65 = local read "Pressure Timeout"() -> (w144:dbl)
        n66 = local read "Trigger Timeout"() -> (w140:dbl)
        n67 = Bundle("Core"=w146, "Pressure Timer"=w147, "Voltage Timer"=w145, "Pressure Timeout"=w144, "Voltage Timeout"=w143, "Display Message"=w142, "Simulate"="Simulate", "Trigger Timeout"=w140, "Trigger Timer"=w139, "Discharge Status Msg"=w138, "scopeTraceGUI::5"=w137, "scopeTraceGUI::7"=w136) -> (w149:T8)  [unwired: 1 in]
        n68 = call <vilib>:"Add State(s) to Queue__jki_lib_state_machine.vi"("State(s) in (\"\")"=w151) -> ("States Out"=w150:string)  [unwired: 14 in]
      }
      frame "Data: Cleanup" {
        # "Cleanup any data and references, here.\n(this is called automatically, by the Macro: Exit)"
        n69 = Unbundle By Name(w152) -> ("Core.Current VI Reference"=w155:refnum<vi>)
        n70 = Close Reference(reference=w155, error in (no error)=w154) -> (error out=w153:errorcluster)
        n71 = call <vilib>:"Add State(s) to Queue__jki_lib_state_machine.vi"("State(s) in (\"\")"=w157) -> ("States Out"=w156:string)  [unwired: 14 in]
      }
      frame "---------- UI ----------" {
        # "Do not put any code in this frame.\n(It is a separator no-op. You can make a copy of this frame to create a new UI frame)"
        n72 = call <vilib>:"Add State(s) to Queue__jki_lib_state_machine.vi"("State(s) in (\"\")"=w161) -> ("States Out"=w160:string)  [unwired: 14 in]
      }
      frame "UI: Initialize" {
        # "Initialize the User Interface, here.\n(this is called automatically, by the Macro: Init)"
        n73 = Unbundle By Name(w163) -> ("Simulate"=w162:bool)
        n74 = case shown="True" w162 {
          frame False {
            w168 = TRUE ("Visible")
            w169 = FALSE ("Visible")
            n75 = property on="Simulate Pressure read" class="DigNum (strict)"("Visible"=w169) -> ()  [unwired: 2 in, 2 out]
            n76 = property on="Simulate voltage" class="DigNum (strict)"("Visible"=w169) -> ()  [unwired: 2 in, 2 out]
            n77 = property on="Simulate Pressure write" class="DigNum (strict)"("Visible"=w169) -> ()  [unwired: 2 in, 2 out]
            n78 = property on="pressure::2" class="DigNum (strict)"("Visible"=w168) -> ()  [unwired: 2 in, 2 out]
            n79 = property on="voltage::3" class="DigNum (strict)"("Visible"=w168) -> ()  [unwired: 2 in, 2 out]
            n80 = property on="Simulate Trig Level" class="DigNum (strict)"("Visible"=w169) -> ()  [unwired: 2 in, 2 out]
          }
          frame True {
            w170 = FALSE ("Visible")
            w171 = TRUE ("Visible")
            n81 = property on="Simulate Pressure read" class="DigNum (strict)"("Visible"=w171) -> ()  [unwired: 2 in, 2 out]
            n82 = property on="Simulate voltage" class="DigNum (strict)"("Visible"=w171) -> ()  [unwired: 2 in, 2 out]
            n83 = property on="Simulate Pressure write" class="DigNum (strict)"("Visible"=w171) -> ()  [unwired: 2 in, 2 out]
            n84 = property on="pressure::2" class="DigNum (strict)"("Visible"=w170) -> ()  [unwired: 2 in, 2 out]
            n85 = property on="voltage::3" class="DigNum (strict)"("Visible"=w170) -> ()  [unwired: 2 in, 2 out]
            n86 = local write "Trigger on"(w170) -> ()
            n87 = property on="Simulate Trig Level" class="DigNum (strict)"("Visible"=w171) -> ()  [unwired: 2 in, 2 out]
          }
        }
        n88 = property on="Display Message" class="Str"("Visible"=FALSE) -> ()  [unwired: 2 in, 2 out]
        n89 = call <vilib>:"Add State(s) to Queue__jki_lib_state_machine.vi"("State(s) in (\"\")"=w167) -> ("States Out"=w166:string)  [unwired: 14 in]
      }
      frame "UI: Cursor Set" {
        # "Argument"
        # "Set and Unset Cursor Busy.\n(Usage: \"UI: Cursor Set >> Busy|Idle\")"
        n90 = case shown="\"Idle\", Default" w172 {
          tunnel: w174 -> [w179 w181]
          tunnel: [w178 w180] -> w173
          frame "Idle", Default {
            n91 = call <vilib>:"Unset Busy.vi"("error in (no error)"=w179) -> ("error out"=w178:errorcluster)  [unwired: 10 in]
          }
          frame "Busy" {
            n92 = call <vilib>:"Set Busy.vi"("error in (no error)"=w181) -> ("error out"=w180:errorcluster)  [unwired: 9 in, 1 out]
          }
        }
        n93 = call <vilib>:"Add State(s) to Queue__jki_lib_state_machine.vi"("State(s) in (\"\")"=w177) -> ("States Out"=w176:string)  [unwired: 14 in]
      }
      frame "UI: Front Panel State" {
        # "Argument"
        # "Set Front Panel Open or Closed\n(Usage: \"UI: Front Panel State >> Open|Close\")"
        n94 = Unbundle By Name(w184) -> ("Core.Current VI Reference"=w183:refnum<vi>)
        n95 = case shown="\"Open\", Default" w182 {
          tunnel: w186 -> [w192 w205]
          tunnel: [w194 w206] -> w185
          tunnel: w183 -> [w193 w203]
          frame "Open", Default {
            n96 = property class="VI"(reference=w193, error in=w192) -> (reference out=w190:refnum<vi>, error out=w191:errorcluster, "Front Panel.Open"=w189:bool)
            n97 = case shown="False" w189 {
              tunnel: [w197 w200] -> w194
              tunnel: w191 -> [w196 w200]
              tunnel: w190 -> [w195 _]
              frame False {
                n98 = invoke class="VI" method="FP.Open"(reference=w195, error in=w196, "Activate"=TRUE, "State"=T6."Standard") -> (error out=w197:errorcluster)  [unwired: 1 in, 4 out]
              }
              frame True {
              }
            }
          }
          frame "Close" {
            n99 = property class="VI"(reference=w203, error in=w205) -> (reference out=w202:refnum<vi>, error out=w204:errorcluster, "Front Panel.Open"=w201:bool)
            n100 = case shown="True" w201 {
              tunnel: [w207 w210] -> w206
              tunnel: w204 -> [w207 w209]
              tunnel: w202 -> [_ w208]
              frame False {
              }
              frame True {
                n101 = invoke class="VI" method="FP.Close"(reference=w208, error in=w209) -> (error out=w210:errorcluster)  [unwired: 1 in, 2 out]
              }
            }
          }
        }
        n102 = call <vilib>:"Add State(s) to Queue__jki_lib_state_machine.vi"("State(s) in (\"\")"=w188) -> ("States Out"=w187:string)  [unwired: 14 in]
      }
      frame "---------- Macro ----------" {
        # "Do not put any code in this frame.\n(It is a separator no-op. You can make a copy of this frame to create a new Macro frame)"
        n103 = call <vilib>:"Add State(s) to Queue__jki_lib_state_machine.vi"("State(s) in (\"\")"=w214) -> ("States Out"=w213:string)  [unwired: 14 in]
      }
      frame "Macro: Initialize" {
        w215 = "Data: Initialize\nInitialize Core Data\nUI: Initialize\nUI: Front Panel State >> Open"  # Data: Initialize Initialize Core Data UI: Initialize UI: Front Panel State >> Open
        # "Initialization Macro\n(This is called once, when the VI starts)"
        n104 = call <vilib>:"Add State(s) to Queue__jki_lib_state_machine.vi"("State(s) in Front (\"\")"=w215, "State(s) in (\"\")"=w219) -> ("States Out"=w218:string)  [unwired: 13 in]
      }
      frame "Macro: Exit" {
        # "Exit Macro\n(This is called once, when the VI exits)"
        n105 = Unbundle By Name(w227) -> ("Core.Close Panel on Exit?"=w226:bool)
        n106 = Select(t="UI: Front Panel State >> Close", s=w226, f="") -> (s? t:f=w223:string)
        n107 = call <vilib>:"Add State(s) to Queue__jki_lib_state_machine.vi"("State(s) in (\"\")"=w223, "State(s) at Back (\"\")"="Data: Cleanup\nExit") -> ("States Out"=w221:string)  [unwired: 13 in]
        n108 = call <vilib>:"Add State(s) to Queue__jki_lib_state_machine.vi"("State(s) in Front (\"\")"=w221, "State(s) in (\"\")"=w229) -> ("States Out"=w228:string)  [unwired: 13 in]
      }
      frame "---------- Start ----------" {
        n109 = call <vilib>:"Add State(s) to Queue__jki_lib_state_machine.vi"("State(s) in (\"\")"=w233) -> ("States Out"=w232:string)  [unwired: 14 in]
      }
      frame "Start: Check Pressure Set point" {
        # "1. check if pressure is \nless than 5"
        n110 = Unbundle By Name(w237) -> ("Pressure Timer"=w238:bool, "Simulate"=w235:bool)
        n111 = case shown="False" w235 {
          tunnel: [w243 w246] -> w234
          frame False {
            n112 = property on="pressure::2" class="DigNum (strict)"() -> ("Value"=w245:dbl)  [unwired: 2 in, 2 out]
            n113 = Greater?(x=w245, y=5.0) -> (0:w243:bool)
          }
          frame True {
            n114 = property on="Simulate Pressure read" class="DigNum (strict)"() -> ("Value"=w247:dbl)  [unwired: 2 in, 2 out]
            n115 = property on="Set Pressure" class="DigNum (strict)"() -> ("Value"=w248:dbl)  [unwired: 2 in, 2 out]
            n116 = call "Calculate limits based on percent tolerance.vi"("Tolerance %"=5.0, "Value"=w248) -> ("Low"=w249:dbl, "High"=w250:dbl)  [unwired: 2 in]
            n117 = In Range and Coerce(upper limit=w250, x=w247, lower limit=w249) -> (In Range?=w246:bool)  [unwired: 1 out]
          }
        }
        n118 = case shown="True" w234 {
          tunnel: [w254 "Start: Check HV"] -> w239
          tunnel: w238 -> [w253 _]
          tunnel: w237 -> [w252 w264]
          tunnel: [w252 w262] -> w236
          frame False {
            n119 = case shown="False" w253 {
              tunnel: ["Start: Set Pressure" w258] -> w254
              frame False {
              }
              frame True {
                n120 = call "Timer.vi"("timer_ops"=timer."Read") -> ("Timer Done?"=w260:bool, "Time Elasped"=→"Time Elasped Pressure":dbl)  [unwired: 2 in, 1 out]
                n121 = Select(t="Error: Pressure Timeout\nDisplay Message>>Pressure Timeout>>Please check pressure settings and devices " ("State(s) in Front (\"\")"), s=w260, f="Start: Check Pressure Set point" ("State(s) in Front (\"\")")) -> (s? t:f=w258:string)
              }
            }
          }
          frame True {
            # "pressure within required range. Check HV settings next"
            # "Start also resets"
            n122 = Bundle By Name(cluster=w264, "Pressure Timer"=FALSE ("Enable Pressure Timer")) -> (w262:T8)
            n123 = call "Timer.vi"("timer_ops"=timer."Start") -> ()  [unwired: 2 in, 3 out]
          }
        }
        n124 = call <vilib>:"Add State(s) to Queue__jki_lib_state_machine.vi"("State(s) in Front (\"\")"=w239, "State(s) in (\"\")"=w242) -> ("States Out"=w241:string)  [unwired: 13 in]
      }
      frame "Stop: Check Pressure Set point" {
        # "1. check if pressure is \nless than 5"
        n125 = Unbundle By Name(w272) -> ("Pressure Timer"=w273:bool, "Simulate"=w270:bool)
        n126 = case shown="False" w270 {
          tunnel: [w278 w279] -> w268
          frame False {
            n127 = property on="pressure::2" class="DigNum (strict)"() -> ("Value"=w278:dbl)  [unwired: 2 in, 2 out]
          }
          frame True {
            n128 = property on="Simulate Pressure read" class="DigNum (strict)"() -> ("Value"=w279:dbl)  [unwired: 2 in, 2 out]
          }
        }
        n129 = Less?(x=w268, y=2.0 ("Tolerance %")) -> (x < y?=w267:bool)
        n130 = case shown="False" w267 {
          tunnel: [w282 "Display Message>>Discharge Is off"] -> w274
          tunnel: w273 -> [w281 _]
          tunnel: w272 -> [w280 w293]
          tunnel: [w280 w291] -> w271
          frame False {
            n131 = case shown="True" w281 {
              tunnel: ["Stop: Set Pressure" w286] -> w282
              frame False {
              }
              frame True {
                n132 = call "Timer.vi"("timer_ops"=timer."Read") -> ("Timer Done?"=w288:bool, "Time Elasped"=→"Time Elasped Pressure 2":dbl)  [unwired: 2 in, 1 out]
                n133 = Select(t="Error: Pressure Timeout\nDisplay Message>>Pressure Timeout>>Please check pressure settings and devices " ("State(s) in Front (\"\")"), s=w288, f="Stop: Check Pressure Set point" ("State(s) in Front (\"\")")) -> (s? t:f=w286:string)
              }
            }
          }
          frame True {
            # "pressure within required range. Check HV settings next"
            # "Start also resets"
            n134 = Bundle By Name(cluster=w293, "Pressure Timer"=FALSE ("Enable Pressure Timer")) -> (w291:T8)
            n135 = call "Timer.vi"("timer_ops"=timer."Start") -> ()  [unwired: 2 in, 3 out]
          }
        }
        n136 = call <vilib>:"Add State(s) to Queue__jki_lib_state_machine.vi"("State(s) in Front (\"\")"=w274, "State(s) in (\"\")"=w277) -> ("States Out"=w276:string)  [unwired: 13 in]
      }
      frame "Start: Set Pressure" {
        n137 = Unbundle By Name(w299) -> ("Pressure Timeout"=w298:dbl, "Simulate"=w295:bool)
        n138 = property on="Set Pressure" class="DigNum (strict)"() -> ("Value"=w297:dbl)  [unwired: 2 in, 2 out]
        n139 = call "Timer.vi"("Timer Value"=w298, "timer_ops"=timer."Start") -> ()  [unwired: 1 in, 3 out]
        n140 = case shown="False" w295 {
          tunnel: w297 -> [w306 w307]
          frame False {
            n141 = property on="Data.Channel 1::1" class="DigNum (strict)"("Val(Sgnl)"=w306) -> ()  [unwired: 2 in, 2 out]
          }
          frame True {
            n142 = property on="Simulate Pressure write" class="DigNum (strict)"("Value"=w307) -> ()  [unwired: 2 in, 2 out]
          }
        }
        n143 = Bundle By Name(cluster=w299, "Pressure Timer"=TRUE ("Enable Pressure Timer")) -> (w301:T8)
        n144 = call <vilib>:"Add State(s) to Queue__jki_lib_state_machine.vi"("State(s) in Front (\"\")"="Display Message>>Changing pressure. Please wait!\nStart: Check Pressure Set point" ("State(s) in Front (\"\")"), "State(s) in (\"\")"=w305) -> ("States Out"=w304:string)  [unwired: 13 in]
      }
      frame "Stop: Set Pressure" {
        n145 = Unbundle By Name(w312) -> ("Pressure Timeout"=w311:dbl, "Simulate"=w309:bool)
        n146 = call "Timer.vi"("Timer Value"=w311, "timer_ops"=timer."Start") -> ()  [unwired: 1 in, 3 out]
        n147 = case shown="False" w309 {
          tunnel: 0.0 ("Value") -> [w319 w320]
          frame False {
            n148 = property on="Data.Channel 1::1" class="DigNum (strict)"("Val(Sgnl)"=w319) -> ()  [unwired: 2 in, 2 out]
          }
          frame True {
            n149 = property on="Simulate Pressure write" class="DigNum (strict)"("Value"=w320) -> ()  [unwired: 2 in, 2 out]
          }
        }
        n150 = Bundle By Name(cluster=w312, "Pressure Timer"=TRUE ("Enable Pressure Timer")) -> (w314:T8)
        n151 = call <vilib>:"Add State(s) to Queue__jki_lib_state_machine.vi"("State(s) in Front (\"\")"="Display Message>>Changing pressure. Please wait!\nStop: Check Pressure Set point" ("State(s) in Front (\"\")"), "State(s) in (\"\")"=w318) -> ("States Out"=w317:string)  [unwired: 13 in]
      }
      frame "Start: Check HV" {
        # "1. check voltage readings\nagainst required voltage"
        n152 = Unbundle By Name(w322) -> ("Voltage Timer"=w324:bool, "Simulate"=w326:bool)
        n153 = case shown="False" w326 {
          tunnel: [w345 w351] -> w325
          frame False {
            n154 = property on="voltage::3" class="DigNum (strict)"() -> ("Value"=w346:dbl)  [unwired: 2 in, 2 out]
            n155 = property on="Set Voltage" class="DigNum (strict)"() -> ("Value"=w350:dbl)  [unwired: 2 in, 2 out]
            n156 = call "Calculate limits based on percent tolerance.vi"("Tolerance %"=5.0, "Value"=w350) -> ("Low"=w347:dbl, "High"=w348:dbl)  [unwired: 2 in]
            n157 = In Range and Coerce(upper limit=w348, x=w346, lower limit=w347) -> (In Range?=w345:bool)  [unwired: 1 out]
          }
          frame True {
            n158 = property on="Simulate voltage" class="DigNum (strict)"() -> ("Value"=w352:dbl)  [unwired: 2 in, 2 out]
            n159 = property on="Set Voltage" class="DigNum (strict)"() -> ("Value"=w353:dbl)  [unwired: 2 in, 2 out]
            n160 = call "Calculate limits based on percent tolerance.vi"("Tolerance %"=5.0, "Value"=w353) -> ("Low"=w355:dbl, "High"=w356:dbl)  [unwired: 2 in]
            n161 = In Range and Coerce(upper limit=w356, x=w352, lower limit=w355) -> (In Range?=w351:bool)  [unwired: 1 out]
          }
        }
        n162 = case shown="False" w325 {
          tunnel: w324 -> [w331 _]
          tunnel: [w332 "Start: Check Trig Level"] -> w323
          tunnel: w322 -> [w330 w343]
          tunnel: [w330 w342] -> w321
          frame False {
            # "2. voltage reading not within range"
            n163 = case shown="True" w331 {
              tunnel: ["Start: Set HV" w336] -> w332
              frame False {
              }
              frame True {
                # "a. check timer and return to \ncurrent state.\nb. dispay error if timer expires"
                n164 = call "Timer.vi"("timer_ops"=timer."Read") -> ("Timer Done?"=w338:bool, "Time Elasped"=→"Time Elasped Voltage":dbl)  [unwired: 2 in, 1 out]
                n165 = Select(t="Error: Voltage Timeout\nDisplay Message>>Voltage Timeout>>Please check Voltage settings and devices ", s=w338, f="Start: Check HV") -> (s? t:f=w336:string)
              }
            }
          }
          frame True {
            # "Start also resets"
            # "The Discharge On"
            n166 = Bundle By Name(cluster=w343, "Voltage Timer"=FALSE) -> (w342:T8)
            n167 = call "Timer.vi"("timer_ops"=timer."Start") -> ()  [unwired: 2 in, 3 out]
          }
        }
        n168 = call <vilib>:"Add State(s) to Queue__jki_lib_state_machine.vi"("State(s) in Front (\"\")"=w323, "State(s) in (\"\")"=w329) -> ("States Out"=w328:string)  [unwired: 13 in]
      }
      frame "Stop: check HV" {
        # "1. check voltage readings\nagainst required voltage"
        n169 = Unbundle By Name(w361) -> ("Voltage Timer"=w363:bool, "Simulate"=w364:bool)
        n170 = case shown="False" w364 {
          tunnel: [w383 w384] -> w359
          frame False {
            n171 = property on="voltage::3" class="DigNum (strict)"() -> ("Value"=w383:dbl)  [unwired: 2 in, 2 out]
          }
          frame True {
            n172 = property on="Simulate voltage" class="DigNum (strict)"() -> ("Value"=w384:dbl)  [unwired: 2 in, 2 out]
          }
        }
        n173 = Less?(x=w359, y=0.5 ("Tolerance %")) -> (x < y?=w357:bool)
        n174 = case shown="True" w357 {
          tunnel: w363 -> [w369 _]
          tunnel: [w370 "Stop: Set Pressure"] -> w362
          tunnel: w361 -> [w368 w381]
          tunnel: [w368 w380] -> w360
          frame False {
            # "2. voltage reading not within range"
            n175 = case shown="True" w369 {
              tunnel: ["Stop: Set HV" w374] -> w370
              frame False {
              }
              frame True {
                # "a. check timer and return to \ncurrent state.\nb. dispay error if timer expires"
                n176 = call "Timer.vi"("timer_ops"=timer."Read") -> ("Timer Done?"=w376:bool, "Time Elasped"=→"Time Elasped Voltage 2":dbl)  [unwired: 2 in, 1 out]
                n177 = Select(t="Error: Voltage Timeout\nDisplay Message>>Voltage Timeout>>Please check Voltage settings and devices ", s=w376, f="Stop: Check HV") -> (s? t:f=w374:string)
              }
            }
          }
          frame True {
            # "Start also resets"
            # "all good. move on"
            n178 = Bundle By Name(cluster=w381, "Voltage Timer"=FALSE) -> (w380:T8)
            n179 = call "Timer.vi"("timer_ops"=timer."Start") -> ()  [unwired: 2 in, 3 out]
          }
        }
        n180 = call <vilib>:"Add State(s) to Queue__jki_lib_state_machine.vi"("State(s) in Front (\"\")"=w362, "State(s) in (\"\")"=w367) -> ("States Out"=w366:string)  [unwired: 13 in]
      }
      frame "Start: set HV" {
        n181 = Unbundle By Name(w389) -> ("Voltage Timeout"=w388:dbl, "Simulate"=w385:bool)
        n182 = call "Timer.vi"("Timer Value"=w388, "timer_ops"=timer."Start") -> ()  [unwired: 1 in, 3 out]
        n183 = property on="Set Voltage" class="DigNum (strict)"() -> ("Value"=w386:dbl)  [unwired: 2 in, 2 out]
        n184 = case shown="False" w385 {
          tunnel: w386 -> [w397 w398]
          frame False {
            n185 = property on="voltage::3" class="DigNum (strict)"("Val(Sgnl)"=w397) -> ()  [unwired: 2 in, 2 out]
          }
          frame True {
            n186 = property on="voltage::3" class="DigNum (strict)"("Value"=w398) -> ()  [unwired: 2 in, 2 out]
          }
        }
        n187 = Bundle By Name(cluster=w389, "Voltage Timer"=TRUE ("Enable Pressure Timer")) -> (w391:T8)
        n188 = disable-structure shown="Disabled" {
          frame Disabled {
            n189 = Wait (ms)(milliseconds to wait=u32 3000) -> ()  [unwired: 1 out]
          }
          frame Enabled {
          }
        }
        n190 = call <vilib>:"Add State(s) to Queue__jki_lib_state_machine.vi"("State(s) in Front (\"\")"="Display Message>>Changing Voltage. Please wait!\nStart: check HV" ("State(s) in Front (\"\")"), "State(s) in (\"\")"=w395) -> ("States Out"=w394:string)  [unwired: 13 in]
      }
      frame "Stop: set HV" {
        n191 = Unbundle By Name(w403) -> ("Voltage Timeout"=w402:dbl, "Simulate"=w400:bool)
        n192 = case shown="True" w400 {
          tunnel: 0.0 ("Value") -> [w410 w411]
          frame False {
            n193 = property on="voltage::3" class="DigNum (strict)"("Val(Sgnl)"=w410) -> ()  [unwired: 2 in, 2 out]
          }
          frame True {
            n194 = property on="voltage::3" class="DigNum (strict)"("Value"=w411) -> ()  [unwired: 2 in, 2 out]
          }
        }
        n195 = call "Timer.vi"("Timer Value"=w402, "timer_ops"=timer."Start") -> ()  [unwired: 1 in, 3 out]
        n196 = Bundle By Name(cluster=w403, "Voltage Timer"=TRUE ("Enable Pressure Timer")) -> (w405:T8)
        n197 = call <vilib>:"Add State(s) to Queue__jki_lib_state_machine.vi"("State(s) in Front (\"\")"="Display Message>>Changing Voltage. Please wait!\nStop: check HV" ("State(s) in Front (\"\")"), "State(s) in (\"\")"=w409) -> ("States Out"=w408:string)  [unwired: 13 in]
      }
      frame "Start: Check Trig Level" {
        # "1. check trig readings\nagainst required voltage"
        n198 = Unbundle By Name(w416) -> ("Trigger Timer"=w419:bool, "Simulate"=w420:bool)
        n199 = local read "Trigger on"() -> (w412:bool)
        n200 = case shown="False" w420 {
          frame False {
          }
          frame True {
          }
        }
        n201 = case shown="False" w412 {
          tunnel: w419 -> [w422 _]
          tunnel: [w423 "Display Message>>Discharge On"] -> w418
          tunnel: w416 -> [w421 w433]
          tunnel: [w421 w432] -> w415
          frame False {
            # "2. trig reading not within range"
            n202 = case shown="True" w422 {
              tunnel: ["Start: Set Trig Level" w427] -> w423
              frame False {
              }
              frame True {
                # "a. check timer and return to \ncurrent state.\nb. dispay error if timer expires"
                n203 = call "Timer.vi"("timer_ops"=timer."Read") -> ("Timer Done?"=w429:bool, "Time Elasped"=→"Time Elasped Trig":dbl)  [unwired: 2 in, 1 out]
                n204 = Select(t="Error: Trigger Timeout\nDisplay Message>>Trigger Timeout>>Please check Trigger settings and devices ", s=w429, f="Start: Check Trig Level") -> (s? t:f=w427:string)
              }
            }
          }
          frame True {
            # "The Discharge On"
            n205 = Bundle By Name(cluster=w433, "Trigger Timer"=FALSE ("Voltage Timer")) -> (w432:T8)
          }
        }
        n206 = call <vilib>:"Add State(s) to Queue__jki_lib_state_machine.vi"("State(s) in Front (\"\")"=w418, "State(s) in (\"\")"=w417) -> ("States Out"=w414:string)  [unwired: 13 in]
      }
      frame "Stop: Check Trig Level" {
        # "1. check trig readings\nagainst required voltage"
        n207 = Unbundle By Name(w439) -> ("Trigger Timer"=w442:bool, "Simulate"=w443:bool)
        n208 = local read "Trigger on"() -> (w435:bool)
        n209 = case shown="True" w443 {
          frame False {
          }
          frame True {
          }
        }
        n210 = case shown="True" w435 {
          tunnel: w442 -> [w445 _]
          tunnel: [w446 "Stop: set HV"] -> w441
          tunnel: w439 -> [w444 w456]
          tunnel: [w444 w455] -> w438
          frame False {
            # "2. trig reading not within range"
            n211 = case shown="True" w445 {
              tunnel: ["Stop: Set Trig Level" w450] -> w446
              frame False {
              }
              frame True {
                # "a. check timer and return to \ncurrent state.\nb. dispay error if timer expires"
                n212 = call "Timer.vi"("timer_ops"=timer."Read") -> ("Timer Done?"=w452:bool, "Time Elasped"=→"Time Elasped Trig 2":dbl)  [unwired: 2 in, 1 out]
                n213 = Select(t="Error: Trigger Timeout\nDisplay Message>>Trigger Timeout>>Please check Trigger settings and devices ", s=w452, f="Stop: Check Trig Level") -> (s? t:f=w450:string)
              }
            }
          }
          frame True {
            # "The Discharge On"
            n214 = Bundle By Name(cluster=w456, "Trigger Timer"=FALSE ("Voltage Timer")) -> (w455:T8)
          }
        }
        n215 = call <vilib>:"Add State(s) to Queue__jki_lib_state_machine.vi"("State(s) in Front (\"\")"=w441, "State(s) in (\"\")"=w440) -> ("States Out"=w437:string)  [unwired: 13 in]
      }
      frame "Start: Set Trig Level" {
        n216 = Unbundle By Name(w460) -> ("Trigger Timeout"=w465:dbl, "Simulate"=w463:bool)
        n217 = call "Timer.vi"("Timer Value"=w465, "timer_ops"=timer."Start") -> ()  [unwired: 1 in, 3 out]
        n218 = case shown="False" w463 {
          frame False {
            n219 = property on="Trigger on" class="Bool (strict)"("Val(Sgnl)"=TRUE ("Channel1.ChannelOn::7")) -> ()  [unwired: 2 in, 2 out]
          }
          frame True {
          }
        }
        n220 = Bundle By Name(cluster=w460, "Trigger Timer"=TRUE ("Enable Pressure Timer")) -> (w459:T8)
        n221 = call <vilib>:"Add State(s) to Queue__jki_lib_state_machine.vi"("State(s) in Front (\"\")"="Display Message>>Changing Trigger Level. Please wait!\nStart: Check Trig Level" ("State(s) in Front (\"\")"), "State(s) in (\"\")"=w462) -> ("States Out"=w461:string)  [unwired: 13 in]
      }
      frame "Stop: Set Trig Level" {
        n222 = Unbundle By Name(w471) -> ("Trigger Timeout"=w476:dbl, "Simulate"=w474:bool)
        n223 = call "Timer.vi"("Timer Value"=w476, "timer_ops"=timer."Start") -> ()  [unwired: 1 in, 3 out]
        n224 = case shown="False" w474 {
          frame False {
            n225 = property on="Trigger on" class="Bool (strict)"("Val(Sgnl)"=FALSE ("Channel1.ChannelOn::7")) -> ()  [unwired: 2 in, 2 out]
          }
          frame True {
          }
        }
        n226 = Bundle By Name(cluster=w471, "Trigger Timer"=TRUE ("Enable Pressure Timer")) -> (w470:T8)
        n227 = call <vilib>:"Add State(s) to Queue__jki_lib_state_machine.vi"("State(s) in Front (\"\")"="Display Message>>Changing Trigger Level. Please wait!\nStop: Check Trig Level" ("State(s) in Front (\"\")"), "State(s) in (\"\")"=w473) -> ("States Out"=w472:string)  [unwired: 13 in]
      }
      frame "Error: Pressure Timeout" {
        n228 = Bundle By Name(cluster=w482, "Pressure Timer"=FALSE ("Enable Pressure Timer")) -> (w481:T8)
        n229 = call <vilib>:"Add State(s) to Queue__jki_lib_state_machine.vi"("State(s) in (\"\")"=w485) -> ("States Out"=w484:string)  [unwired: 14 in]
      }
      frame "Error: Voltage Timeout" {
        n230 = Bundle By Name(cluster=w488, "Voltage Timer"=FALSE ("Enable Pressure Timer")) -> (w487:T8)
        n231 = call <vilib>:"Add State(s) to Queue__jki_lib_state_machine.vi"("State(s) in (\"\")"=w491) -> ("States Out"=w490:string)  [unwired: 14 in]
      }
      frame "Error: Trigger Timeout" {
        n232 = Bundle By Name(cluster=w494, "Trigger Timer"=FALSE ("Enable Pressure Timer")) -> (w493:T8)
        n233 = call <vilib>:"Add State(s) to Queue__jki_lib_state_machine.vi"("State(s) in (\"\")"=w497) -> ("States Out"=w496:string)  [unwired: 14 in]
      }
      frame "Display Message" {
        n234 = property on="Display Message" class="Str"("Visible"=TRUE, "Value"=w500) -> ()  [unwired: 2 in, 2 out]
        n235 = call <userlib>:"String to 1D Array__ogtk.vi"("delimiter (Tab)"=">>", "string"=w500) -> ()  [unwired: 9 in, 1 out]
        n236 = call <vilib>:"Add State(s) to Queue__jki_lib_state_machine.vi"("State(s) in (\"\")"=w504) -> ("States Out"=w503:string)  [unwired: 14 in]
      }
      frame "update2" {
        n237 = Unbundle By Name(w507) -> ("Simulate"=w537:bool)
        n238 = case shown="False" w537 {
          tunnel: [w557 w572] -> w522
          tunnel: [w556 w569] -> w509
          tunnel: [_ w568] -> w508
          frame True {
            n239 = property on="Set Pressure" class="DigNum (strict)"() -> ("Value"=w564:dbl)  [unwired: 2 in, 2 out]
            n240 = property on="Set Voltage" class="DigNum (strict)"() -> ("Value"=w563:dbl)  [unwired: 2 in, 2 out]
            n241 = property on="Simulate Pressure read" class="DigNum (strict)"() -> ("Value"=w558:dbl)  [unwired: 2 in, 2 out]
            n242 = property on="Simulate voltage" class="DigNum (strict)"() -> ("Value"=w559:dbl)  [unwired: 2 in, 2 out]
            n243 = call "Calculate limits based on percent tolerance.vi"("Tolerance %"=5.0, "Value"=w563) -> ("Low"=w560:dbl, "High"=w561:dbl)  [unwired: 2 in]
            n244 = call "Calculate limits based on percent tolerance.vi"("Tolerance %"=5.0, "Value"=w564) -> ("Low"=w565:dbl, "High"=w566:dbl)  [unwired: 2 in]
            n245 = In Range and Coerce(upper limit=w566, x=w558, lower limit=w565) -> (In Range?=w556:bool)  [unwired: 1 out]
            n246 = In Range and Coerce(upper limit=w561, x=w559, lower limit=w560) -> (In Range?=w557:bool)  [unwired: 1 out]
          }
          frame False {
            n247 = property on="pressure::2" class="DigNum (strict)"() -> ("Value"=w570:dbl)  [unwired: 2 in, 2 out]
            n248 = property on="voltage::3" class="DigNum (strict)"() -> ("Value"=w574:dbl)  [unwired: 2 in, 2 out]
            n249 = local read "Trigger on"() -> (w568:bool)
            n250 = Greater?(x=w574, y=5.0) -> (0:w572:bool)
            n251 = Greater?(x=w570, y=1.5) -> (0:w569:bool)
          }
        }
        n252 = case shown="\"in\"" "position::6" {
          tunnel: [u32 13816530 u32 16318208 u32 16711680] -> w514
          frame "out", Default {
          }
          frame "Unknown" {
          }
          frame "in" {
          }
        }
        n253 = property on="position::6" class="Enum (strict)"("RingText.FG Color"=w514, "RingText.BGColor"=w514) -> ()  [unwired: 2 in, 2 out]
        n254 = local read "Trigger on"() -> (w505:bool)
        n255 = Compound Arithmetic op=AND(w522, w508, w509) -> (w513:bool)
        n256 = Not(x=w513) -> (.not. x?=w510:bool)
        n257 = And(x=w510, y="Enable cap interlock move out") -> (x .and. y?=w512:bool)
        n258 = case "stop triggers if voltage or P not good" shown="True" w512 {
          tunnel: "position::6" -> [_ w545]
          tunnel: w505 -> [_ w544]
          frame False {
          }
          frame True {
            n259 = case shown="True" w544 {
              frame False {
              }
              frame True {
                n260 = property on="Trigger on" class="Bool (strict)"("Val(Sgnl)"=FALSE ("Channel1.ChannelOn::7")) -> ()  [unwired: 2 in, 2 out]
              }
            }
            n261 = case shown="\"in\", Default" w545 {
              frame "out" {
              }
              frame "in", Default {
                n262 = property on="position::6" class="Enum (strict)"("Val(Sgnl)"=enum16{"out", "in", "Unknown"}."out" ("Value (Signaling)")) -> ()  [unwired: 2 in, 2 out]
                n263 = Wait (ms)(milliseconds to wait=u32 1000) -> ()  [unwired: 1 out]
              }
            }
          }
        }
        n264 = Select(t="Discharge On", s=w513, f="Discharge Off") -> (s? t:f=w521:string)
        n265 = Bundle By Name(cluster=w507, "Discharge Status Msg"=w521) -> ()  [unwired: 1 out]
        n266 = Select(t=u32 6618880, s=w513, f=u32 16711680) -> (s? t:f=w532:u32)
        n267 = case shown="False" "Force button visibility" {
          tunnel: [w551 TRUE ("Visible")] -> w518
          tunnel: [w550 TRUE] -> w517
          tunnel: w513 -> [w550 _]
          tunnel: "position::6" -> [w549 _]
          frame False {
            n268 = case shown="\"in\", Default" w549 {
              tunnel: [TRUE ("Visible") FALSE ("Visible")] -> w551
              frame "out" {
              }
              frame "in", Default {
              }
            }
          }
          frame True {
          }
        }
        n269 = property on="Discharge Status Msg" class="Str"("Value"=w521, "Text.BGColor"=w532) -> ()  [unwired: 2 in, 2 out]
        n270 = property on="position::6" class="Enum (strict)"("Visible"=w517) -> ()  [unwired: 2 in, 2 out]
        n271 = property on="Start/Stop discharge" class="Bool (strict)"("Visible"=w518) -> ()  [unwired: 2 in, 2 out]
        n272 = Select(t="", s=w522, f="Display Message>>Please check voltage settings and devices ") -> (s? t:f=w529:string)
        n273 = Not(x=w522) -> (.not. x?=w526:bool)
        n274 = Not(x=w509) -> (.not. x?=w527:bool)
        n275 = Select(t=w529, s=w509, f="Display Message>>Please check pressure settings and devices ") -> (s? t:f=w523:string)
        n276 = And(x=w526, y=w527) -> (x .and. y?=w525:bool)
        n277 = Select(t="Display Message>>Please check voltage and pressure (settings and devices )", s=w525, f=w523) -> (s? t:f=w520:string)
        n278 = Concatenate Strings(w520, "\ndigitizer traces") -> (w506:string)
        n279 = call <vilib>:"Add State(s) to Queue__jki_lib_state_machine.vi"("State(s) in Front (\"\")"=w506, "State(s) in (\"\")"=w540) -> ("States Out"=w539:string)  [unwired: 13 in]
      }
      frame "update1" {
        n280 = Greater?(x="amplitude.Channel_C::10", y=0.2) -> (0:w575:bool)
        n281 = local write "Trigger on"(w575) -> ()
        n282 = call <vilib>:"Add State(s) to Queue__jki_lib_state_machine.vi"("State(s) in (\"\")"=w581) -> ("States Out"=w580:string)  [unwired: 14 in]
      }
      frame "duplicateme" {
        n283 = call <vilib>:"Add State(s) to Queue__jki_lib_state_machine.vi"("State(s) in (\"\")"=w585) -> ("States Out"=w584:string)  [unwired: 14 in]
      }
      frame "digitizer traces" {
        (unwired) waveform(dbl)[] [] ("scopeTraceGUI::5")
        (unwired) waveform(dbl) {"t0"=timestamp(0 s since 1904-01-01), "dt"=1.0, "Y"=[]} ("Waveform")
        n284 = Unbundle By Name("Digitizer Traces") -> ("scopeTraceGUI::5"=w591:waveform(dbl)[])
        n285 = Unbundle By Name(w594) -> ("scopeTraceGUI::5"=w595:waveform(dbl)[])
        n286 = Not Equal?(x=w595, y=w591) -> (x != y?=w593:bool)
        n287 = Index Array(array=w591) -> (element=w590:waveform(dbl))  [unwired: 1 in]
        n288 = call-poly <vilib>:"Waveform Duration.vi"("waveform in"=w590) -> ("duration"=w589:dbl)  [unwired: 8 in, 2 out]
        "duration" <- w589
        n289 = Greater Than 0?(x=w589) -> (x > 0?=w588:bool)
        n290 = Compound Arithmetic op=AND(w593, w588) -> (w592:bool)
        n291 = case shown="True" w592 {
          tunnel: [w601 w612] -> w596
          tunnel: w591 -> [_ w610]
          tunnel: w594 -> [w601 w611]
          tunnel: w587 -> [w600 w608]
          tunnel: [w600 w607] -> w586
          frame False {
          }
          frame True {
            n292 = Build Array("value3::9", "value4::9", "value5::9", "value6::9") -> (w602:dbl[])
            n293 = for {
              tunnel: w610 -> [w616] mode=indexing
              tunnel: w602 -> [w614] mode=indexing
              tunnel: [w618] -> w609 mode=indexing
              tunnel: w608 -> [w617]
              tunnel: [w617] -> w607
              n294 = Unbundle By Name(w616) -> ("t0"=w615:timestamp)
              n295 = Add(x=w615, y=w614) -> (x+y=w613:timestamp)
              n296 = Bundle By Name(cluster=w616, "t0"=w613) -> (w618:waveform(dbl))
            }
            "all traces" <- w609
            n297 = Bundle By Name(cluster=w611, "scopeTraceGUI::5"=w609) -> (w612:T8)
          }
        }
        n298 = call <vilib>:"Add State(s) to Queue__jki_lib_state_machine.vi"("State(s) in (\"\")"=w599) -> ("States Out"=w598:string)  [unwired: 14 in]
      }
    }
  }
  n299 = call "GUI_Master_subvi_reentrant_queues.vi"("STOP Queue in"=w3, "This Application"=w9, "error in (no error)"=w10, "tcp data event"=w8, "Caller menu reference"=w12, "Caller VI ref"=w13) -> ("error out"=→"error IO 2":errorcluster)  [unwired: 5 in]
  n300 = call <userlib>:"Fit VI window to Largest Dec__ogtk.vi"() -> ()  [unwired: 6 in, 2 out]
  n301 = disable-structure shown="Disabled" {
    frame Disabled {
      n302 = property on="Start/Stop discharge" class="Bool (strict)" props=["Visible"]() -> ()  [unwired: 3 in, 2 out]
    }
    frame Enabled {
    }
  }
  n303 = Unregister For Events(event registration refnum=w4, error in=w1) -> (error out=w2:errorcluster)
  n304 = Release Queue(queue=w3, error in (no error)=w1) -> ()  [unwired: 1 in, 3 out]
  n305 = Destroy User Event(user event=w8, error in=w2) -> ()  [unwired: 1 out]
